vi "compress_discretes_fast_1.vi"(6 "DI state table":T1[](array[typedef]), 8 "discret parameters":bool[](array[boolean]), 9 "DI table":string[](array[string]), 10 "date/time string":string, 11 "table":string) -> (2 "Data to write":bool, 3 "parameters":string)   [LabVIEW 2019, in "PostgreSQL.lvlib"]
uses:
  PostgreSQL.lvlib
  Inputs/Ctl/Parameter State.ctl
  Inputs/Inputs.lvlib
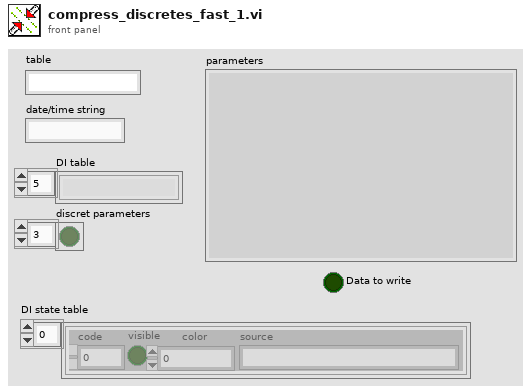
[diagram p1: front panel]
types:
  T1 = typedef "Inputs.lvlib/Parameter State.ctl" = cluster{"code":i32, "visible":bool, "color":u32, "source":string}
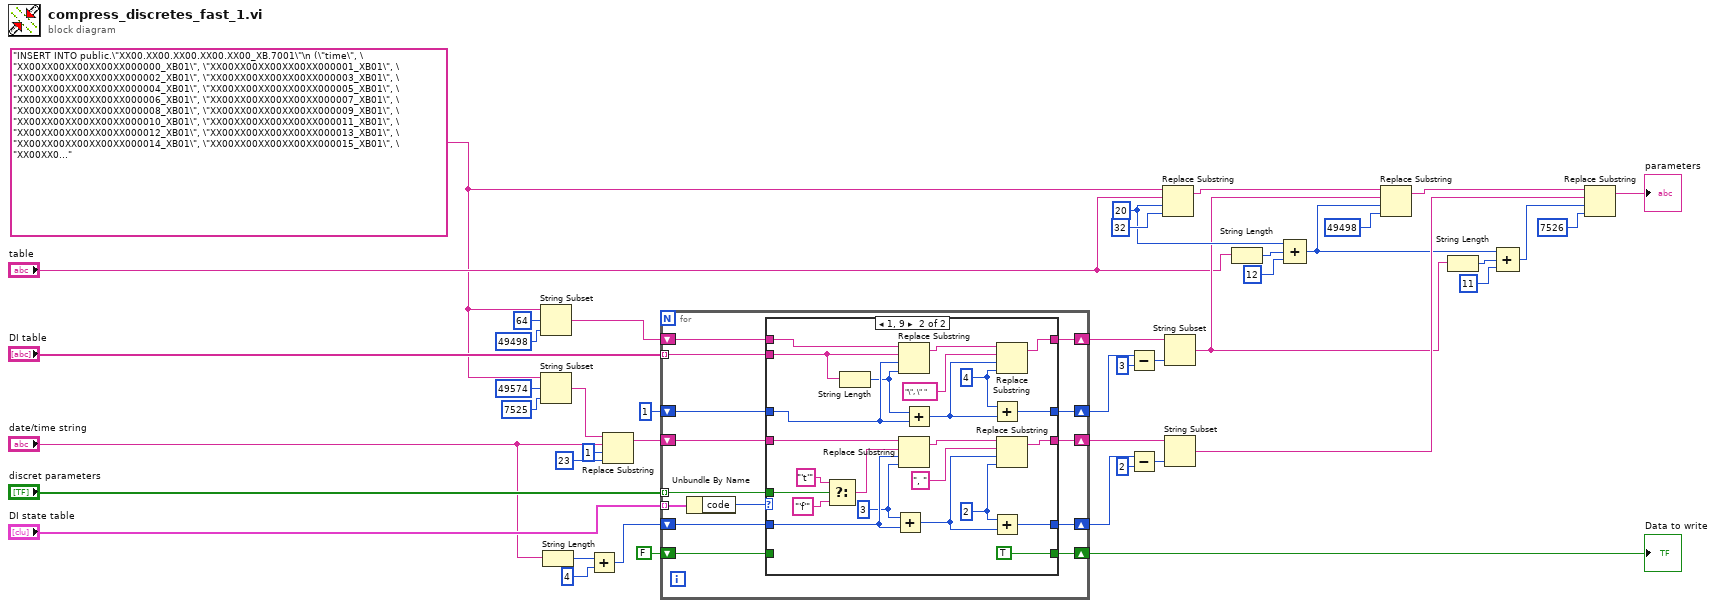
[diagram p0: block diagram]
diagram:
  w32 = 20 ("offset (0)")
  w10 = "INSERT INTO public.\"XX00.XX00.XX00.XX00.XX00_XB.7001\"\n (\"time\", \"XX00XX00XX00XX00XX000000_XB01\", \"XX00XX00XX00XX00XX000001_XB01\", \"XX00XX00XX00XX00XX000002_XB01\", \"XX00XX00XX00XX00XX000003_XB01\", \"XX00XX00XX00XX00XX000004_XB01\", \"XX00XX00XX00XX00XX000005_XB01\", \"XX00XX00XX00XX00XX000006_XB01\", \"XX00XX00XX00XX00XX000007_XB01\", \"XX00XX00XX00XX00XX000008_XB01\", \"XX00XX00XX00XX00XX000009_XB01\", \"XX00XX00XX00XX00XX000010_XB01\", \"XX00XX00XX00XX00XX000011_XB01\", \"XX00XX00XX00XX00XX000012_XB01\", \"XX00XX00XX00XX00XX000013_XB01\", \"XX00XX00XX00XX00XX000014_XB01\", \"XX00XX00XX00XX00XX000015_XB01\", \"XX00XX00XX00XX00XX000016_XB01\", \"XX00XX00XX00XX00XX000017_XB01\", \"XX00XX00XX00XX00XX000018_XB01\", \"XX00XX00XX00XX00XX000019_XB01\", \"XX00XX00XX00XX00XX000020_XB01\", \"XX00XX00XX00XX00XX000021_XB01\", \"XX00XX00XX00XX00XX000022_XB01\", \"XX00XX00XX00XX00XX000023_XB01\", \"XX00XX00XX00XX00XX000024_XB01\", \"XX00XX00XX00XX00XX000025_XB01\", \"XX00XX00XX00XX00XX000026_XB01\", \"XX00XX00XX00XX00XX000027_XB01\", \"XX00XX00XX00XX00XX000028_XB01\", \"XX00XX00XX00XX00XX000029_XB01\", \"XX00XX00XX00XX00XX000030_XB01\", \"XX00XX00XX00XX00XX000031_XB01\", \"XX00XX00XX00XX00XX000032_XB01\", \"XX00XX00XX00XX00XX000033_XB01\", \"XX00XX00XX00XX00XX000034_XB01\", \"XX00XX00XX00XX00XX000035_XB01\", \"XX00XX00XX00XX00XX000036_XB01\", \"XX00XX00XX00XX00XX000037_XB01\", \"XX00XX00XX00XX00XX000038_XB01\", \"XX00XX00XX00XX00XX000039_XB01\", \"XX00XX00XX00XX00XX000040_XB01\", \"XX00XX00XX00XX00XX000041_XB01\", \"XX00XX00XX00XX00XX000042_XB01\", \"XX00XX00XX00XX00XX000043_XB01\", \"XX00XX00XX00XX00XX000044_XB01\", \"XX00XX00XX00XX00XX000045_XB01\", \"XX00XX00XX00XX00XX000046_XB01\", \"XX00XX00XX00XX00XX000047_XB01\", \"XX00XX00XX00XX00XX000048_XB01\", \"XX00XX00XX00XX00XX000049_XB01\", \"XX00XX00XX00XX00XX000050_XB01\", \"XX00XX00XX00XX00XX000051_XB01\", \"XX00XX00XX00XX00XX000052_XB01\", \"XX00XX00XX00XX00XX000053_XB01\", \"XX00XX00XX00XX00XX000054_XB01\", \"XX00XX00XX00XX00XX000055_XB01\", \"XX00XX00XX00XX00XX000056_XB01\", \"XX00XX00XX00XX00XX000057_XB01\", \"XX00XX00XX00XX00XX000058_XB01\", \"XX00XX00XX00XX00XX000059_XB01\", \"XX00XX00XX00XX00XX000060_XB01\", \"XX00XX00XX00XX00XX000061_XB01\", \"XX00XX00XX00XX00XX000062_XB01\", \"XX00XX00XX00XX00XX000063_XB01\", \"XX00XX00XX00XX00XX000064_XB01\", \"XX00XX00XX00XX00XX000065_XB01\", \"XX00XX00XX00XX00XX000066_XB01\", \"XX00XX00XX00XX00XX000067_XB01\", \"XX00XX00XX00XX00XX000068_XB01\", \"XX00XX00XX00XX00XX000069_XB01\", \"XX00XX00XX00XX00XX000070_XB01\", \"XX00XX00XX00XX00XX000071_XB01\", \"XX00XX00XX00XX00XX000072_XB01\", \"XX00XX00XX00XX00XX000073_XB01\", \"XX00XX00XX00XX00XX000074_XB01\", \"XX00XX00XX00XX00XX000075_XB01\", \"XX00XX00XX00XX00XX000076_XB01\", \"XX00XX00XX00XX00XX000077_XB01\", \"XX00XX00XX00XX00XX000078_XB01\", \"XX00XX00XX00XX00XX000079_XB01\", \"XX00XX00XX00XX00XX000080_XB01\", \"XX00XX00XX00XX00XX000081_XB01\", \"XX00XX00XX00XX00XX000082_XB01\", \"XX00XX00XX00XX00XX000083_XB01\", \"XX00XX00XX00XX00XX000084_XB01\", \"XX00XX00XX00XX00XX000085_XB01\", \"XX00XX00XX00XX00XX000086_XB01\", \"XX00XX00XX00XX00XX000087_XB01\", \"XX00XX00XX00XX00XX000088_XB01\", \"XX00XX00XX00XX00XX000089_XB01\", \"XX00XX00XX00XX00XX000090_XB01\", \"XX00XX00XX00XX00XX000091_XB01\", \"XX00XX00XX00XX00XX000092_XB01\", \"XX00XX00XX00XX00XX000093_XB01\", \"XX00XX00XX00XX00XX000094_XB01\", \"XX00XX00XX00XX00XX000095_XB01\", \"XX00XX00XX00XX00XX000096_XB01\", \"XX00XX00XX00XX00XX000097_XB01\", \"XX00XX00XX00XX00XX000098_XB01\", \"XX00XX00XX00XX00XX000099_XB01\", \"XX00XX00XX00XX00XX000100_XB01\", \"XX00XX00XX00XX00XX000101_XB01\", \"XX00XX00XX00XX00XX000102_XB01\", \"XX00XX00XX00XX00XX000103_XB01\", \"XX00XX00XX00XX00XX000104_XB01\", \"XX00XX00XX00XX00XX000105_XB01\", \"XX00XX00XX00XX00XX000106_XB01\", \"XX00XX00XX00XX00XX000107_XB01\", \"XX00XX00XX00XX00XX000108_XB01\", \"XX00XX00XX00XX00XX000109_XB01\", \"XX00XX00XX00XX00XX000110_XB01\", \"XX00XX00XX00XX00XX000111_XB01\", \"XX00XX00XX00XX00XX000112_XB01\", \"XX00XX00XX00XX00XX000113_XB01\", \"XX00XX00XX00XX00XX000114_XB01\", \"XX00XX00XX00XX00XX000115_XB01\", \"XX00XX00XX00XX00XX000116_XB01\", \"XX00XX00XX00XX00XX000117_XB01\", \"XX00XX00XX00XX00XX000118_XB01\", \"XX00XX00XX00XX00XX000119_XB01\", \"XX00XX00XX00XX00XX000120_XB01\", \"XX00XX00XX00XX00XX000121_XB01\", \"XX00XX00XX00XX00XX000122_XB01\", \"XX00XX00XX00XX00XX000123_XB01\", \"XX00XX00XX00XX00XX000124_XB01\", \"XX00XX00XX00XX00XX000125_XB01\", \"XX00XX00XX00XX00XX000126_XB01\", \"XX00XX00XX00XX00XX000127_XB01\", \"XX00XX00XX00XX00XX000128_XB01\", \"XX00XX00XX00XX00XX000129_XB01\", \"XX00XX00XX00XX00XX000130_XB01\", \"XX00XX00XX00XX00XX000131_XB01\", \"XX00XX00XX00XX00XX000132_XB01\", \"XX00XX00XX00XX00XX000133_XB01\", \"XX00XX00XX00XX00XX000134_XB01\", \"XX00XX00XX00XX00XX000135_XB01\", \"XX00XX00XX00XX00XX000136_XB01\", \"XX00XX00XX00XX00XX000137_XB01\", \"XX00XX00XX00XX00XX000138_XB01\", \"XX00XX00XX00XX00XX000139_XB01\", \"XX00XX00XX00XX00XX000140_XB01\", \"XX00XX00XX00XX00XX000141_XB01\", \"XX00XX00XX00XX00XX000142_XB01\", \"XX00XX00XX00XX00XX000143_XB01\", \"XX00XX00XX00XX00XX000144_XB01\", \"XX00XX00XX00XX00XX000145_XB01\", \"XX00XX00XX00XX00XX000146_XB01\", \"XX00XX00XX00XX00XX000147_XB01\", \"XX00XX00XX00XX00XX000148_XB01\", \"XX00XX00XX00XX00XX000149_XB01\", \"XX00XX00XX00XX00XX000150_XB01\", \"XX00XX00XX00XX00XX000151_XB01\", \"XX00XX00XX00XX00XX000152_XB01\", \"XX00XX00XX00XX00XX000153_XB01\", \"XX00XX00XX00XX00XX000154_XB01\", \"XX00XX00XX00XX00XX000155_XB01\", \"XX00XX00XX00XX00XX000156_XB01\", \"XX00XX00XX00XX00XX000157_XB01\", \"XX00XX00XX00XX00XX000158_XB01\", \"XX00XX00XX00XX00XX000159_XB01\", \"XX00XX00XX00XX00XX000160_XB01\", \"XX00XX00XX00XX00XX000161_XB01\", \"XX00XX00XX00XX00XX000162_XB01\", \"XX00XX00XX00XX00XX000163_XB01\", \"XX00XX00XX00XX00XX000164_XB01\", \"XX00XX00XX00XX00XX000165_XB01\", \"XX00XX00XX00XX00XX000166_XB01\", \"XX00XX00XX00XX00XX000167_XB01\", \"XX00XX00XX00XX00XX000168_XB01\", \"XX00XX00XX00XX00XX000169_XB01\", \"XX00XX00XX00XX00XX000170_XB01\", \"XX00XX00XX00XX00XX000171_XB01\", \"XX00XX00XX00XX00XX000172_XB01\", \"XX00XX00XX00XX00XX000173_XB01\", \"XX00XX00XX00XX00XX000174_XB01\", \"XX00XX00XX00XX00XX000175_XB01\", \"XX00XX00XX00XX00XX000176_XB01\", \"XX00XX00XX00XX00XX000177_XB01\", \"XX00XX00XX00XX00XX000178_XB01\", \"XX00XX00XX00XX00XX000179_XB01\", \"XX00XX00XX00XX00XX000180_XB01\", \"XX00XX00XX00XX00XX000181_XB01\", \"XX00XX00XX00XX00XX000182_XB01\", \"XX00XX00XX00XX00XX000183_XB01\", \"XX00XX00XX00XX00XX000184_XB01\", \"XX00XX00XX00XX00XX000185_XB01\", \"XX00XX00XX00XX00XX000186_XB01\", \"XX00XX00XX00XX00XX000187_XB01\", \"XX00XX00XX00XX00XX000188_XB01\", \"XX00XX00XX00XX00XX000189_XB01\", \"XX00XX00XX00XX00XX000190_XB01\", \"XX00XX00XX00XX00XX000191_XB01\", \"XX00XX00XX00XX00XX000192_XB01\", \"XX00XX00XX00XX00XX000193_XB01\", \"XX00XX00XX00XX00XX000194_XB01\", \"XX00XX00XX00XX00XX000195_XB01\", \"XX00XX00XX00XX00XX000196_XB01\", \"XX00XX00XX00XX00XX000197_XB01\", \"XX00XX00XX00XX00XX000198_XB01\", \"XX00XX00XX00XX00XX000199_XB01\", \"XX00XX00XX00XX00XX000200_XB01\", \"XX00XX00XX00XX00XX000201_XB01\", \"XX00XX00XX00XX00XX000202_XB01\", \"XX00XX00XX00XX00XX000203_XB01\", \"XX00XX00XX00XX00XX000204_XB01\", \"XX00XX00XX00XX00XX000205_XB01\", \"XX00XX00XX00XX00XX000206_XB01\", \"XX00XX00XX00XX00XX000207_XB01\", \"XX00XX00XX00XX00XX000208_XB01\", \"XX00XX00XX00XX00XX000209_XB01\", \"XX00XX00XX00XX00XX000210_XB01\", \"XX00XX00XX00XX00XX000211_XB01\", \"XX00XX00XX00XX00XX000212_XB01\", \"XX00XX00XX00XX00XX000213_XB01\", \"XX00XX00XX00XX00XX000214_XB01\", \"XX00XX00XX00XX00XX000215_XB01\", \"XX00XX00XX00XX00XX000216_XB01\", \"XX00XX00XX00XX00XX000217_XB01\", \"XX00XX00XX00XX00XX000218_XB01\", \"XX00XX00XX00XX00XX000219_XB01\", \"XX00XX00XX00XX00XX000220_XB01\", \"XX00XX00XX00XX00XX000221_XB01\", \"XX00XX00XX00XX00XX000222_XB01\", \"XX00XX00XX00XX00XX000223_XB01\", \"XX00XX00XX00XX00XX000224_XB01\", \"XX00XX00XX00XX00XX000225_XB01\", \"XX00XX00XX00XX00XX000226_XB01\", \"XX00XX00XX00XX00XX000227_XB01\", \"XX00XX00XX00XX00XX000228_XB01\", \"XX00XX00XX00XX00XX000229_XB01\", \"XX00XX00XX00XX00XX000230_XB01\", \"XX00XX00XX00XX00XX000231_XB01\", \"XX00XX00XX00XX00XX000232_XB01\", \"XX00XX00XX00XX00XX000233_XB01\", \"XX00XX00XX00XX00XX000234_XB01\", \"XX00XX00XX00XX00XX000235_XB01\", \"XX00XX00XX00XX00XX000236_XB01\", \"XX00XX00XX00XX00XX000237_XB01\", \"XX00XX00XX00XX00XX000238_XB01\", \"XX00XX00XX00XX00XX000239_XB01\", \"XX00XX00XX00XX00XX000240_XB01\", \"XX00XX00XX00XX00XX000241_XB01\", \"XX00XX00XX00XX00XX000242_XB01\", \"XX00XX00XX00XX00XX000243_XB01\", \"XX00XX00XX00XX00XX000244_XB01\", \"XX00XX00XX00XX00XX000245_XB01\", \"XX00XX00XX00XX00XX000246_XB01\", \"XX00XX00XX00XX00XX000247_XB01\", \"XX00XX00XX00XX00XX000248_XB01\", \"XX00XX00XX00XX00XX000249_XB01\", \"XX00XX00XX00XX00XX000250_XB01\", \"XX00XX00XX00XX00XX000251_XB01\", \"XX00XX00XX00XX00XX000252_XB01\", \"XX00XX00XX00XX00XX000253_XB01\", \"XX00XX00XX00XX00XX000254_XB01\", \"XX00XX00XX00XX00XX000255_XB01\", \"XX00XX00XX00XX00XX000256_XB01\", \"XX00XX00XX00XX00XX000257_XB01\", \"XX00XX00XX00XX00XX000258_XB01\", \"XX00XX00XX00XX00XX000259_XB01\", \"XX00XX00XX00XX00XX000260_XB01\", \"XX00XX00XX00XX00XX000261_XB01\", \"XX00XX00XX00XX00XX000262_XB01\", \"XX00XX00XX00XX00XX000263_XB01\", \"XX00XX00XX00XX00XX000264_XB01\", \"XX00XX00XX00XX00XX000265_XB01\", \"XX00XX00XX00XX00XX000266_XB01\", \"XX00XX00XX00XX00XX000267_XB01\", \"XX00XX00XX00XX00XX000268_XB01\", \"XX00XX00XX00XX00XX000269_XB01\", \"XX00XX00XX00XX00XX000270_XB01\", \"XX00XX00XX00XX00XX000271_XB01\", \"XX00XX00XX00XX00XX000272_XB01\", \"XX00XX00XX00XX00XX000273_XB01\", \"XX00XX00XX00XX00XX000274_XB01\", \"XX00XX00XX00XX00XX000275_XB01\", \"XX00XX00XX00XX00XX000276_XB01\", \"XX00XX00XX00XX00XX000277_XB01\", \"XX00XX00XX00XX00XX000278_XB01\", \"XX00XX00XX00XX00XX000279_XB01\", \"XX00XX00XX00XX00XX000280_XB01\", \"XX00XX00XX00XX00XX000281_XB01\", \"XX00XX00XX00XX00XX000282_XB01\", \"XX00XX00XX00XX00XX000283_XB01\", \"XX00XX00XX00XX00XX000284_XB01\", \"XX00XX00XX00XX00XX000285_XB01\", \"XX00XX00XX00XX00XX000286_XB01\", \"XX00XX00XX00XX00XX000287_XB01\", \"XX00XX00XX00XX00XX000288_XB01\", \"XX00XX00XX00XX00XX000289_XB01\", \"XX00XX00XX00XX00XX000290_XB01\", \"XX00XX00XX00XX00XX000291_XB01\", \"XX00XX00XX00XX00XX000292_XB01\", \"XX00XX00XX00XX00XX000293_XB01\", \"XX00XX00XX00XX00XX000294_XB01\", \"XX00XX00XX00XX00XX000295_XB01\", \"XX00XX00XX00XX00XX000296_XB01\", \"XX00XX00XX00XX00XX000297_XB01\", \"XX00XX00XX00XX00XX000298_XB01\", \"XX00XX00XX00XX00XX000299_XB01\", \"XX00XX00XX00XX00XX000300_XB01\", \"XX00XX00XX00XX00XX000301_XB01\", \"XX00XX00XX00XX00XX000302_XB01\", \"XX00XX00XX00XX00XX000303_XB01\", \"XX00XX00XX00XX00XX000304_XB01\", \"XX00XX00XX00XX00XX000305_XB01\", \"XX00XX00XX00XX00XX000306_XB01\", \"XX00XX00XX00XX00XX000307_XB01\", \"XX00XX00XX00XX00XX000308_XB01\", \"XX00XX00XX00XX00XX000309_XB01\", \"XX00XX00XX00XX00XX000310_XB01\", \"XX00XX00XX00XX00XX000311_XB01\", \"XX00XX00XX00XX00XX000312_XB01\", \"XX00XX00XX00XX00XX000313_XB01\", \"XX00XX00XX00XX00XX000314_XB01\", \"XX00XX00XX00XX00XX000315_XB01\", \"XX00XX00XX00XX00XX000316_XB01\", \"XX00XX00XX00XX00XX000317_XB01\", \"XX00XX00XX00XX00XX000318_XB01\", \"XX00XX00XX00XX00XX000319_XB01\", \"XX00XX00XX00XX00XX000320_XB01\", \"XX00XX00XX00XX00XX000321_XB01\", \"XX00XX00XX00XX00XX000322_XB01\", \"XX00XX00XX00XX00XX000323_XB01\", \"XX00XX00XX00XX00XX000324_XB01\", \"XX00XX00XX00XX00XX000325_XB01\", \"XX00XX00XX00XX00XX000326_XB01\", \"XX00XX00XX00XX00XX000327_XB01\", \"XX00XX00XX00XX00XX000328_XB01\", \"XX00XX00XX00XX00XX000329_XB01\", \"XX00XX00XX00XX00XX000330_XB01\", \"XX00XX00XX00XX00XX000331_XB01\", \"XX00XX00XX00XX00XX000332_XB01\", \"XX00XX00XX00XX00XX000333_XB01\", \"XX00XX00XX00XX00XX000334_XB01\", \"XX00XX00XX00XX00XX000335_XB01\", \"XX00XX00XX00XX00XX000336_XB01\", \"XX00XX00XX00XX00XX000337_XB01\", \"XX00XX00XX00XX00XX000338_XB01\", \"XX00XX00XX00XX00XX000339_XB01\", \"XX00XX00XX00XX00XX000340_XB01\", \"XX00XX00XX00XX00XX000341_XB01\", \"XX00XX00XX00XX00XX000342_XB01\", \"XX00XX00XX00XX00XX000343_XB01\", \"XX00XX00XX00XX00XX000344_XB01\", \"XX00XX00XX00XX00XX000345_XB01\", \"XX00XX00XX00XX00XX000346_XB01\", \"XX00XX00XX00XX00XX000347_XB01\", \"XX00XX00XX00XX00XX000348_XB01\", \"XX00XX00XX00XX00XX000349_XB01\", \"XX00XX00XX00XX00XX000350_XB01\", \"XX00XX00XX00XX00XX000351_XB01\", \"XX00XX00XX00XX00XX000352_XB01\", \"XX00XX00XX00XX00XX000353_XB01\", \"XX00XX00XX00XX00XX000354_XB01\", \"XX00XX00XX00XX00XX000355_XB01\", \"XX00XX00XX00XX00XX000356_XB01\", \"XX00XX00XX00XX00XX000357_XB01\", \"XX00XX00XX00XX00XX000358_XB01\", \"XX00XX00XX00XX00XX000359_XB01\", \"XX00XX00XX00XX00XX000360_XB01\", \"XX00XX00XX00XX00XX000361_XB01\", \"XX00XX00XX00XX00XX000362_XB01\", \"XX00XX00XX00XX00XX000363_XB01\", \"XX00XX00XX00XX00XX000364_XB01\", \"XX00XX00XX00XX00XX000365_XB01\", \"XX00XX00XX00XX00XX000366_XB01\", \"XX00XX00XX00XX00XX000367_XB01\", \"XX00XX00XX00XX00XX000368_XB01\", \"XX00XX00XX00XX00XX000369_XB01\", \"XX00XX00XX00XX00XX000370_XB01\", \"XX00XX00XX00XX00XX000371_XB01\", \"XX00XX00XX00XX00XX000372_XB01\", \"XX00XX00XX00XX00XX000373_XB01\", \"XX00XX00XX00XX00XX000374_XB01\", \"XX00XX00XX00XX00XX000375_XB01\", \"XX00XX00XX00XX00XX000376_XB01\", \"XX00XX00XX00XX00XX000377_XB01\", \"XX00XX00XX00XX00XX000378_XB01\", \"XX00XX00XX00XX00XX000379_XB01\", \"XX00XX00XX00XX00XX000380_XB01\", \"XX00XX00XX00XX00XX000381_XB01\", \"XX00XX00XX00XX00XX000382_XB01\", \"XX00XX00XX00XX00XX000383_XB01\", \"XX00XX00XX00XX00XX000384_XB01\", \"XX00XX00XX00XX00XX000385_XB01\", \"XX00XX00XX00XX00XX000386_XB01\", \"XX00XX00XX00XX00XX000387_XB01\", \"XX00XX00XX00XX00XX000388_XB01\", \"XX00XX00XX00XX00XX000389_XB01\", \"XX00XX00XX00XX00XX000390_XB01\", \"XX00XX00XX00XX00XX000391_XB01\", \"XX00XX00XX00XX00XX000392_XB01\", \"XX00XX00XX00XX00XX000393_XB01\", \"XX00XX00XX00XX00XX000394_XB01\", \"XX00XX00XX00XX00XX000395_XB01\", \"XX00XX00XX00XX00XX000396_XB01\", \"XX00XX00XX00XX00XX000397_XB01\", \"XX00XX00XX00XX00XX000398_XB01\", \"XX00XX00XX00XX00XX000399_XB01\", \"XX00XX00XX00XX00XX000400_XB01\", \"XX00XX00XX00XX00XX000401_XB01\", \"XX00XX00XX00XX00XX000402_XB01\", \"XX00XX00XX00XX00XX000403_XB01\", \"XX00XX00XX00XX00XX000404_XB01\", \"XX00XX00XX00XX00XX000405_XB01\", \"XX00XX00XX00XX00XX000406_XB01\", \"XX00XX00XX00XX00XX000407_XB01\", \"XX00XX00XX00XX00XX000408_XB01\", \"XX00XX00XX00XX00XX000409_XB01\", \"XX00XX00XX00XX00XX000410_XB01\", \"XX00XX00XX00XX00XX000411_XB01\", \"XX00XX00XX00XX00XX000412_XB01\", \"XX00XX00XX00XX00XX000413_XB01\", \"XX00XX00XX00XX00XX000414_XB01\", \"XX00XX00XX00XX00XX000415_XB01\", \"XX00XX00XX00XX00XX000416_XB01\", \"XX00XX00XX00XX00XX000417_XB01\", \"XX00XX00XX00XX00XX000418_XB01\", \"XX00XX00XX00XX00XX000419_XB01\", \"XX00XX00XX00XX00XX000420_XB01\", \"XX00XX00XX00XX00XX000421_XB01\", \"XX00XX00XX00XX00XX000422_XB01\", \"XX00XX00XX00XX00XX000423_XB01\", \"XX00XX00XX00XX00XX000424_XB01\", \"XX00XX00XX00XX00XX000425_XB01\", \"XX00XX00XX00XX00XX000426_XB01\", \"XX00XX00XX00XX00XX000427_XB01\", \"XX00XX00XX00XX00XX000428_XB01\", \"XX00XX00XX00XX00XX000429_XB01\", \"XX00XX00XX00XX00XX000430_XB01\", \"XX00XX00XX00XX00XX000431_XB01\", \"XX00XX00XX00XX00XX000432_XB01\", \"XX00XX00XX00XX00XX000433_XB01\", \"XX00XX00XX00XX00XX000434_XB01\", \"XX00XX00XX00XX00XX000435_XB01\", \"XX00XX00XX00XX00XX000436_XB01\", \"XX00XX00XX00XX00XX000437_XB01\", \"XX00XX00XX00XX00XX000438_XB01\", \"XX00XX00XX00XX00XX000439_XB01\", \"XX00XX00XX00XX00XX000440_XB01\", \"XX00XX00XX00XX00XX000441_XB01\", \"XX00XX00XX00XX00XX000442_XB01\", \"XX00XX00XX00XX00XX000443_XB01\", \"XX00XX00XX00XX00XX000444_XB01\", \"XX00XX00XX00XX00XX000445_XB01\", \"XX00XX00XX00XX00XX000446_XB01\", \"XX00XX00XX00XX00XX000447_XB01\", \"XX00XX00XX00XX00XX000448_XB01\", \"XX00XX00XX00XX00XX000449_XB01\", \"XX00XX00XX00XX00XX000450_XB01\", \"XX00XX00XX00XX00XX000451_XB01\", \"XX00XX00XX00XX00XX000452_XB01\", \"XX00XX00XX00XX00XX000453_XB01\", \"XX00XX00XX00XX00XX000454_XB01\", \"XX00XX00XX00XX00XX000455_XB01\", \"XX00XX00XX00XX00XX000456_XB01\", \"XX00XX00XX00XX00XX000457_XB01\", \"XX00XX00XX00XX00XX000458_XB01\", \"XX00XX00XX00XX00XX000459_XB01\", \"XX00XX00XX00XX00XX000460_XB01\", \"XX00XX00XX00XX00XX000461_XB01\", \"XX00XX00XX00XX00XX000462_XB01\", \"XX00XX00XX00XX00XX000463_XB01\", \"XX00XX00XX00XX00XX000464_XB01\", \"XX00XX00XX00XX00XX000465_XB01\", \"XX00XX00XX00XX00XX000466_XB01\", \"XX00XX00XX00XX00XX000467_XB01\", \"XX00XX00XX00XX00XX000468_XB01\", \"XX00XX00XX00XX00XX000469_XB01\", \"XX00XX00XX00XX00XX000470_XB01\", \"XX00XX00XX00XX00XX000471_XB01\", \"XX00XX00XX00XX00XX000472_XB01\", \"XX00XX00XX00XX00XX000473_XB01\", \"XX00XX00XX00XX00XX000474_XB01\", \"XX00XX00XX00XX00XX000475_XB01\", \"XX00XX00XX00XX00XX000476_XB01\", \"XX00XX00XX00XX00XX000477_XB01\", \"XX00XX00XX00XX00XX000478_XB01\", \"XX00XX00XX00XX00XX000479_XB01\", \"XX00XX00XX00XX00XX000480_XB01\", \"XX00XX00XX00XX00XX000481_XB01\", \"XX00XX00XX00XX00XX000482_XB01\", \"XX00XX00XX00XX00XX000483_XB01\", \"XX00XX00XX00XX00XX000484_XB01\", \"XX00XX00XX00XX00XX000485_XB01\", \"XX00XX00XX00XX00XX000486_XB01\", \"XX00XX00XX00XX00XX000487_XB01\", \"XX00XX00XX00XX00XX000488_XB01\", \"XX00XX00XX00XX00XX000489_XB01\", \"XX00XX00XX00XX00XX000490_XB01\", \"XX00XX00XX00XX00XX000491_XB01\", \"XX00XX00XX00XX00XX000492_XB01\", \"XX00XX00XX00XX00XX000493_XB01\", \"XX00XX00XX00XX00XX000494_XB01\", \"XX00XX00XX00XX00XX000495_XB01\", \"XX00XX00XX00XX00XX000496_XB01\", \"XX00XX00XX00XX00XX000497_XB01\", \"XX00XX00XX00XX00XX000498_XB01\", \"XX00XX00XX00XX00XX000499_XB01\", \"XX00XX00XX00XX00XX000500_XB01\", \"XX00XX00XX00XX00XX000501_XB01\", \"XX00XX00XX00XX00XX000502_XB01\", \"XX00XX00XX00XX00XX000503_XB01\", \"XX00XX00XX00XX00XX000504_XB01\", \"XX00XX00XX00XX00XX000505_XB01\", \"XX00XX00XX00XX00XX000506_XB01\", \"XX00XX00XX00XX00XX000507_XB01\", \"XX00XX00XX00XX00XX000508_XB01\", \"XX00XX00XX00XX00XX000509_XB01\", \"XX00XX00XX00XX00XX000510_XB01\", \"XX00XX00XX00XX00XX000511_XB01\", \"XX00XX00XX00XX00XX000512_XB01\", \"XX00XX00XX00XX00XX000513_XB01\", \"XX00XX00XX00XX00XX000514_XB01\", \"XX00XX00XX00XX00XX000515_XB01\", \"XX00XX00XX00XX00XX000516_XB01\", \"XX00XX00XX00XX00XX000517_XB01\", \"XX00XX00XX00XX00XX000518_XB01\", \"XX00XX00XX00XX00XX000519_XB01\", \"XX00XX00XX00XX00XX000520_XB01\", \"XX00XX00XX00XX00XX000521_XB01\", \"XX00XX00XX00XX00XX000522_XB01\", \"XX00XX00XX00XX00XX000523_XB01\", \"XX00XX00XX00XX00XX000524_XB01\", \"XX00XX00XX00XX00XX000525_XB01\", \"XX00XX00XX00XX00XX000526_XB01\", \"XX00XX00XX00XX00XX000527_XB01\", \"XX00XX00XX00XX00XX000528_XB01\", \"XX00XX00XX00XX00XX000529_XB01\", \"XX00XX00XX00XX00XX000530_XB01\", \"XX00XX00XX00XX00XX000531_XB01\", \"XX00XX00XX00XX00XX000532_XB01\", \"XX00XX00XX00XX00XX000533_XB01\", \"XX00XX00XX00XX00XX000534_XB01\", \"XX00XX00XX00XX00XX000535_XB01\", \"XX00XX00XX00XX00XX000536_XB01\", \"XX00XX00XX00XX00XX000537_XB01\", \"XX00XX00XX00XX00XX000538_XB01\", \"XX00XX00XX00XX00XX000539_XB01\", \"XX00XX00XX00XX00XX000540_XB01\", \"XX00XX00XX00XX00XX000541_XB01\", \"XX00XX00XX00XX00XX000542_XB01\", \"XX00XX00XX00XX00XX000543_XB01\", \"XX00XX00XX00XX00XX000544_XB01\", \"XX00XX00XX00XX00XX000545_XB01\", \"XX00XX00XX00XX00XX000546_XB01\", \"XX00XX00XX00XX00XX000547_XB01\", \"XX00XX00XX00XX00XX000548_XB01\", \"XX00XX00XX00XX00XX000549_XB01\", \"XX00XX00XX00XX00XX000550_XB01\", \"XX00XX00XX00XX00XX000551_XB01\", \"XX00XX00XX00XX00XX000552_XB01\", \"XX00XX00XX00XX00XX000553_XB01\", \"XX00XX00XX00XX00XX000554_XB01\", \"XX00XX00XX00XX00XX000555_XB01\", \"XX00XX00XX00XX00XX000556_XB01\", \"XX00XX00XX00XX00XX000557_XB01\", \"XX00XX00XX00XX00XX000558_XB01\", \"XX00XX00XX00XX00XX000559_XB01\", \"XX00XX00XX00XX00XX000560_XB01\", \"XX00XX00XX00XX00XX000561_XB01\", \"XX00XX00XX00XX00XX000562_XB01\", \"XX00XX00XX00XX00XX000563_XB01\", \"XX00XX00XX00XX00XX000564_XB01\", \"XX00XX00XX00XX00XX000565_XB01\", \"XX00XX00XX00XX00XX000566_XB01\", \"XX00XX00XX00XX00XX000567_XB01\", \"XX00XX00XX00XX00XX000568_XB01\", \"XX00XX00XX00XX00XX000569_XB01\", \"XX00XX00XX00XX00XX000570_XB01\", \"XX00XX00XX00XX00XX000571_XB01\", \"XX00XX00XX00XX00XX000572_XB01\", \"XX00XX00XX00XX00XX000573_XB01\", \"XX00XX00XX00XX00XX000574_XB01\", \"XX00XX00XX00XX00XX000575_XB01\", \"XX00XX00XX00XX00XX000576_XB01\", \"XX00XX00XX00XX00XX000577_XB01\", \"XX00XX00XX00XX00XX000578_XB01\", \"XX00XX00XX00XX00XX000579_XB01\", \"XX00XX00XX00XX00XX000580_XB01\", \"XX00XX00XX00XX00XX000581_XB01\", \"XX00XX00XX00XX00XX000582_XB01\", \"XX00XX00XX00XX00XX000583_XB01\", \"XX00XX00XX00XX00XX000584_XB01\", \"XX00XX00XX00XX00XX000585_XB01\", \"XX00XX00XX00XX00XX000586_XB01\", \"XX00XX00XX00XX00XX000587_XB01\", \"XX00XX00XX00XX00XX000588_XB01\", \"XX00XX00XX00XX00XX000589_XB01\", \"XX00XX00XX00XX00XX000590_XB01\", \"XX00XX00XX00XX00XX000591_XB01\", \"XX00XX00XX00XX00XX000592_XB01\", \"XX00XX00XX00XX00XX000593_XB01\", \"XX00XX00XX00XX00XX000594_XB01\", \"XX00XX00XX00XX00XX000595_XB01\", \"XX00XX00XX00XX00XX000596_XB01\", \"XX00XX00XX00XX00XX000597_XB01\", \"XX00XX00XX00XX00XX000598_XB01\", \"XX00XX00XX00XX00XX000599_XB01\", \"XX00XX00XX00XX00XX000600_XB01\", \"XX00XX00XX00XX00XX000601_XB01\", \"XX00XX00XX00XX00XX000602_XB01\", \"XX00XX00XX00XX00XX000603_XB01\", \"XX00XX00XX00XX00XX000604_XB01\", \"XX00XX00XX00XX00XX000605_XB01\", \"XX00XX00XX00XX00XX000606_XB01\", \"XX00XX00XX00XX00XX000607_XB01\", \"XX00XX00XX00XX00XX000608_XB01\", \"XX00XX00XX00XX00XX000609_XB01\", \"XX00XX00XX00XX00XX000610_XB01\", \"XX00XX00XX00XX00XX000611_XB01\", \"XX00XX00XX00XX00XX000612_XB01\", \"XX00XX00XX00XX00XX000613_XB01\", \"XX00XX00XX00XX00XX000614_XB01\", \"XX00XX00XX00XX00XX000615_XB01\", \"XX00XX00XX00XX00XX000616_XB01\", \"XX00XX00XX00XX00XX000617_XB01\", \"XX00XX00XX00XX00XX000618_XB01\", \"XX00XX00XX00XX00XX000619_XB01\", \"XX00XX00XX00XX00XX000620_XB01\", \"XX00XX00XX00XX00XX000621_XB01\", \"XX00XX00XX00XX00XX000622_XB01\", \"XX00XX00XX00XX00XX000623_XB01\", \"XX00XX00XX00XX00XX000624_XB01\", \"XX00XX00XX00XX00XX000625_XB01\", \"XX00XX00XX00XX00XX000626_XB01\", \"XX00XX00XX00XX00XX000627_XB01\", \"XX00XX00XX00XX00XX000628_XB01\", \"XX00XX00XX00XX00XX000629_XB01\", \"XX00XX00XX00XX00XX000630_XB01\", \"XX00XX00XX00XX00XX000631_XB01\", \"XX00XX00XX00XX00XX000632_XB01\", \"XX00XX00XX00XX00XX000633_XB01\", \"XX00XX00XX00XX00XX000634_XB01\", \"XX00XX00XX00XX00XX000635_XB01\", \"XX00XX00XX00XX00XX000636_XB01\", \"XX00XX00XX00XX00XX000637_XB01\", \"XX00XX00XX00XX00XX000638_XB01\", \"XX00XX00XX00XX00XX000639_XB01\", \"XX00XX00XX00XX00XX000640_XB01\", \"XX00XX00XX00XX00XX000641_XB01\", \"XX00XX00XX00XX00XX000642_XB01\", \"XX00XX00XX00XX00XX000643_XB01\", \"XX00XX00XX00XX00XX000644_XB01\", \"XX00XX00XX00XX00XX000645_XB01\", \"XX00XX00XX00XX00XX000646_XB01\", \"XX00XX00XX00XX00XX000647_XB01\", \"XX00XX00XX00XX00XX000648_XB01\", \"XX00XX00XX00XX00XX000649_XB01\", \"XX00XX00XX00XX00XX000650_XB01\", \"XX00XX00XX00XX00XX000651_XB01\", \"XX00XX00XX00XX00XX000652_XB01\", \"XX00XX00XX00XX00XX000653_XB01\", \"XX00XX00XX00XX00XX000654_XB01\", \"XX00XX00XX00XX00XX000655_XB01\", \"XX00XX00XX00XX00XX000656_XB01\", \"XX00XX00XX00XX00XX000657_XB01\", \"XX00XX00XX00XX00XX000658_XB01\", \"XX00XX00XX00XX00XX000659_XB01\", \"XX00XX00XX00XX00XX000660_XB01\", \"XX00XX00XX00XX00XX000661_XB01\", \"XX00XX00XX00XX00XX000662_XB01\", \"XX00XX00XX00XX00XX000663_XB01\", \"XX00XX00XX00XX00XX000664_XB01\", \"XX00XX00XX00XX00XX000665_XB01\", \"XX00XX00XX00XX00XX000666_XB01\", \"XX00XX00XX00XX00XX000667_XB01\", \"XX00XX00XX00XX00XX000668_XB01\", \"XX00XX00XX00XX00XX000669_XB01\", \"XX00XX00XX00XX00XX000670_XB01\", \"XX00XX00XX00XX00XX000671_XB01\", \"XX00XX00XX00XX00XX000672_XB01\", \"XX00XX00XX00XX00XX000673_XB01\", \"XX00XX00XX00XX00XX000674_XB01\", \"XX00XX00XX00XX00XX000675_XB01\", \"XX00XX00XX00XX00XX000676_XB01\", \"XX00XX00XX00XX00XX000677_XB01\", \"XX00XX00XX00XX00XX000678_XB01\", \"XX00XX00XX00XX00XX000679_XB01\", \"XX00XX00XX00XX00XX000680_XB01\", \"XX00XX00XX00XX00XX000681_XB01\", \"XX00XX00XX00XX00XX000682_XB01\", \"XX00XX00XX00XX00XX000683_XB01\", \"XX00XX00XX00XX00XX000684_XB01\", \"XX00XX00XX00XX00XX000685_XB01\", \"XX00XX00XX00XX00XX000686_XB01\", \"XX00XX00XX00XX00XX000687_XB01\", \"XX00XX00XX00XX00XX000688_XB01\", \"XX00XX00XX00XX00XX000689_XB01\", \"XX00XX00XX00XX00XX000690_XB01\", \"XX00XX00XX00XX00XX000691_XB01\", \"XX00XX00XX00XX00XX000692_XB01\", \"XX00XX00XX00XX00XX000693_XB01\", \"XX00XX00XX00XX00XX000694_XB01\", \"XX00XX00XX00XX00XX000695_XB01\", \"XX00XX00XX00XX00XX000696_XB01\", \"XX00XX00XX00XX00XX000697_XB01\", \"XX00XX00XX00XX00XX000698_XB01\", \"XX00XX00XX00XX00XX000699_XB01\", \"XX00XX00XX00XX00XX000700_XB01\", \"XX00XX00XX00XX00XX000701_XB01\", \"XX00XX00XX00XX00XX000702_XB01\", \"XX00XX00XX00XX00XX000703_XB01\", \"XX00XX00XX00XX00XX000704_XB01\", \"XX00XX00XX00XX00XX000705_XB01\", \"XX00XX00XX00XX00XX000706_XB01\", \"XX00XX00XX00XX00XX000707_XB01\", \"XX00XX00XX00XX00XX000708_XB01\", \"XX00XX00XX00XX00XX000709_XB01\", \"XX00XX00XX00XX00XX000710_XB01\", \"XX00XX00XX00XX00XX000711_XB01\", \"XX00XX00XX00XX00XX000712_XB01\", \"XX00XX00XX00XX00XX000713_XB01\", \"XX00XX00XX00XX00XX000714_XB01\", \"XX00XX00XX00XX00XX000715_XB01\", \"XX00XX00XX00XX00XX000716_XB01\", \"XX00XX00XX00XX00XX000717_XB01\", \"XX00XX00XX00XX00XX000718_XB01\", \"XX00XX00XX00XX00XX000719_XB01\", \"XX00XX00XX00XX00XX000720_XB01\", \"XX00XX00XX00XX00XX000721_XB01\", \"XX00XX00XX00XX00XX000722_XB01\", \"XX00XX00XX00XX00XX000723_XB01\", \"XX00XX00XX00XX00XX000724_XB01\", \"XX00XX00XX00XX00XX000725_XB01\", \"XX00XX00XX00XX00XX000726_XB01\", \"XX00XX00XX00XX00XX000727_XB01\", \"XX00XX00XX00XX00XX000728_XB01\", \"XX00XX00XX00XX00XX000729_XB01\", \"XX00XX00XX00XX00XX000730_XB01\", \"XX00XX00XX00XX00XX000731_XB01\", \"XX00XX00XX00XX00XX000732_XB01\", \"XX00XX00XX00XX00XX000733_XB01\", \"XX00XX00XX00XX00XX000734_XB01\", \"XX00XX00XX00XX00XX000735_XB01\", \"XX00XX00XX00XX00XX000736_XB01\", \"XX00XX00XX00XX00XX000737_XB01\", \"XX00XX00XX00XX00XX000738_XB01\", \"XX00XX00XX00XX00XX000739_XB01\", \"XX00XX00XX00XX00XX000740_XB01\", \"XX00XX00XX00XX00XX000741_XB01\", \"XX00XX00XX00XX00XX000742_XB01\", \"XX00XX00XX00XX00XX000743_XB01\", \"XX00XX00XX00XX00XX000744_XB01\", \"XX00XX00XX00XX00XX000745_XB01\", \"XX00XX00XX00XX00XX000746_XB01\", \"XX00XX00XX00XX00XX000747_XB01\", \"XX00XX00XX00XX00XX000748_XB01\", \"XX00XX00XX00XX00XX000749_XB01\", \"XX00XX00XX00XX00XX000750_XB01\", \"XX00XX00XX00XX00XX000751_XB01\", \"XX00XX00XX00XX00XX000752_XB01\", \"XX00XX00XX00XX00XX000753_XB01\", \"XX00XX00XX00XX00XX000754_XB01\", \"XX00XX00XX00XX00XX000755_XB01\", \"XX00XX00XX00XX00XX000756_XB01\", \"XX00XX00XX00XX00XX000757_XB01\", \"XX00XX00XX00XX00XX000758_XB01\", \"XX00XX00XX00XX00XX000759_XB01\", \"XX00XX00XX00XX00XX000760_XB01\", \"XX00XX00XX00XX00XX000761_XB01\", \"XX00XX00XX00XX00XX000762_XB01\", \"XX00XX00XX00XX00XX000763_XB01\", \"XX00XX00XX00XX00XX000764_XB01\", \"XX00XX00XX00XX00XX000765_XB01\", \"XX00XX00XX00XX00XX000766_XB01\", \"XX00XX00XX00XX00XX000767_XB01\", \"XX00XX00XX00XX00XX000768_XB01\", \"XX00XX00XX00XX00XX000769_XB01\", \"XX00XX00XX00XX00XX000770_XB01\", \"XX00XX00XX00XX00XX000771_XB01\", \"XX00XX00XX00XX00XX000772_XB01\", \"XX00XX00XX00XX00XX000773_XB01\", \"XX00XX00XX00XX00XX000774_XB01\", \"XX00XX00XX00XX00XX000775_XB01\", \"XX00XX00XX00XX00XX000776_XB01\", \"XX00XX00XX00XX00XX000777_XB01\", \"XX00XX00XX00XX00XX000778_XB01\", \"XX00XX00XX00XX00XX000779_XB01\", \"XX00XX00XX00XX00XX000780_XB01\", \"XX00XX00XX00XX00XX000781_XB01\", \"XX00XX00XX00XX00XX000782_XB01\", \"XX00XX00XX00XX00XX000783_XB01\", \"XX00XX00XX00XX00XX000784_XB01\", \"XX00XX00XX00XX00XX000785_XB01\", \"XX00XX00XX00XX00XX000786_XB01\", \"XX00XX00XX00XX00XX000787_XB01\", \"XX00XX00XX00XX00XX000788_XB01\", \"XX00XX00XX00XX00XX000789_XB01\", \"XX00XX00XX00XX00XX000790_XB01\", \"XX00XX00XX00XX00XX000791_XB01\", \"XX00XX00XX00XX00XX000792_XB01\", \"XX00XX00XX00XX00XX000793_XB01\", \"XX00XX00XX00XX00XX000794_XB01\", \"XX00XX00XX00XX00XX000795_XB01\", \"XX00XX00XX00XX00XX000796_XB01\", \"XX00XX00XX00XX00XX000797_XB01\", \"XX00XX00XX00XX00XX000798_XB01\", \"XX00XX00XX00XX00XX000799_XB01\", \"XX00XX00XX00XX00XX000800_XB01\", \"XX00XX00XX00XX00XX000801_XB01\", \"XX00XX00XX00XX00XX000802_XB01\", \"XX00XX00XX00XX00XX000803_XB01\", \"XX00XX00XX00XX00XX000804_XB01\", \"XX00XX00XX00XX00XX000805_XB01\", \"XX00XX00XX00XX00XX000806_XB01\", \"XX00XX00XX00XX00XX000807_XB01\", \"XX00XX00XX00XX00XX000808_XB01\", \"XX00XX00XX00XX00XX000809_XB01\", \"XX00XX00XX00XX00XX000810_XB01\", \"XX00XX00XX00XX00XX000811_XB01\", \"XX00XX00XX00XX00XX000812_XB01\", \"XX00XX00XX00XX00XX000813_XB01\", \"XX00XX00XX00XX00XX000814_XB01\", \"XX00XX00XX00XX00XX000815_XB01\", \"XX00XX00XX00XX00XX000816_XB01\", \"XX00XX00XX00XX00XX000817_XB01\", \"XX00XX00XX00XX00XX000818_XB01\", \"XX00XX00XX00XX00XX000819_XB01\", \"XX00XX00XX00XX00XX000820_XB01\", \"XX00XX00XX00XX00XX000821_XB01\", \"XX00XX00XX00XX00XX000822_XB01\", \"XX00XX00XX00XX00XX000823_XB01\", \"XX00XX00XX00XX00XX000824_XB01\", \"XX00XX00XX00XX00XX000825_XB01\", \"XX00XX00XX00XX00XX000826_XB01\", \"XX00XX00XX00XX00XX000827_XB01\", \"XX00XX00XX00XX00XX000828_XB01\", \"XX00XX00XX00XX00XX000829_XB01\", \"XX00XX00XX00XX00XX000830_XB01\", \"XX00XX00XX00XX00XX000831_XB01\", \"XX00XX00XX00XX00XX000832_XB01\", \"XX00XX00XX00XX00XX000833_XB01\", \"XX00XX00XX00XX00XX000834_XB01\", \"XX00XX00XX00XX00XX000835_XB01\", \"XX00XX00XX00XX00XX000836_XB01\", \"XX00XX00XX00XX00XX000837_XB01\", \"XX00XX00XX00XX00XX000838_XB01\", \"XX00XX00XX00XX00XX000839_XB01\", \"XX00XX00XX00XX00XX000840_XB01\", \"XX00XX00XX00XX00XX000841_XB01\", \"XX00XX00XX00XX00XX000842_XB01\", \"XX00XX00XX00XX00XX000843_XB01\", \"XX00XX00XX00XX00XX000844_XB01\", \"XX00XX00XX00XX00XX000845_XB01\", \"XX00XX00XX00XX00XX000846_XB01\", \"XX00XX00XX00XX00XX000847_XB01\", \"XX00XX00XX00XX00XX000848_XB01\", \"XX00XX00XX00XX00XX000849_XB01\", \"XX00XX00XX00XX00XX000850_XB01\", \"XX00XX00XX00XX00XX000851_XB01\", \"XX00XX00XX00XX00XX000852_XB01\", \"XX00XX00XX00XX00XX000853_XB01\", \"XX00XX00XX00XX00XX000854_XB01\", \"XX00XX00XX00XX00XX000855_XB01\", \"XX00XX00XX00XX00XX000856_XB01\", \"XX00XX00XX00XX00XX000857_XB01\", \"XX00XX00XX00XX00XX000858_XB01\", \"XX00XX00XX00XX00XX000859_XB01\", \"XX00XX00XX00XX00XX000860_XB01\", \"XX00XX00XX00XX00XX000861_XB01\", \"XX00XX00XX00XX00XX000862_XB01\", \"XX00XX00XX00XX00XX000863_XB01\", \"XX00XX00XX00XX00XX000864_XB01\", \"XX00XX00XX00XX00XX000865_XB01\", \"XX00XX00XX00XX00XX000866_XB01\", \"XX00XX00XX00XX00XX000867_XB01\", \"XX00XX00XX00XX00XX000868_XB01\", \"XX00XX00XX00XX00XX000869_XB01\", \"XX00XX00XX00XX00XX000870_XB01\", \"XX00XX00XX00XX00XX000871_XB01\", \"XX00XX00XX00XX00XX000872_XB01\", \"XX00XX00XX00XX00XX000873_XB01\", \"XX00XX00XX00XX00XX000874_XB01\", \"XX00XX00XX00XX00XX000875_XB01\", \"XX00XX00XX00XX00XX000876_XB01\", \"XX00XX00XX00XX00XX000877_XB01\", \"XX00XX00XX00XX00XX000878_XB01\", \"XX00XX00XX00XX00XX000879_XB01\", \"XX00XX00XX00XX00XX000880_XB01\", \"XX00XX00XX00XX00XX000881_XB01\", \"XX00XX00XX00XX00XX000882_XB01\", \"XX00XX00XX00XX00XX000883_XB01\", \"XX00XX00XX00XX00XX000884_XB01\", \"XX00XX00XX00XX00XX000885_XB01\", \"XX00XX00XX00XX00XX000886_XB01\", \"XX00XX00XX00XX00XX000887_XB01\", \"XX00XX00XX00XX00XX000888_XB01\", \"XX00XX00XX00XX00XX000889_XB01\", \"XX00XX00XX00XX00XX000890_XB01\", \"XX00XX00XX00XX00XX000891_XB01\", \"XX00XX00XX00XX00XX000892_XB01\", \"XX00XX00XX00XX00XX000893_XB01\", \"XX00XX00XX00XX00XX000894_XB01\", \"XX00XX00XX00XX00XX000895_XB01\", \"XX00XX00XX00XX00XX000896_XB01\", \"XX00XX00XX00XX00XX000897_XB01\", \"XX00XX00XX00XX00XX000898_XB01\", \"XX00XX00XX00XX00XX000899_XB01\", \"XX00XX00XX00XX00XX000900_XB01\", \"XX00XX00XX00XX00XX000901_XB01\", \"XX00XX00XX00XX00XX000902_XB01\", \"XX00XX00XX00XX00XX000903_XB01\", \"XX00XX00XX00XX00XX000904_XB01\", \"XX00XX00XX00XX00XX000905_XB01\", \"XX00XX00XX00XX00XX000906_XB01\", \"XX00XX00XX00XX00XX000907_XB01\", \"XX00XX00XX00XX00XX000908_XB01\", \"XX00XX00XX00XX00XX000909_XB01\", \"XX00XX00XX00XX00XX000910_XB01\", \"XX00XX00XX00XX00XX000911_XB01\", \"XX00XX00XX00XX00XX000912_XB01\", \"XX00XX00XX00XX00XX000913_XB01\", \"XX00XX00XX00XX00XX000914_XB01\", \"XX00XX00XX00XX00XX000915_XB01\", \"XX00XX00XX00XX00XX000916_XB01\", \"XX00XX00XX00XX00XX000917_XB01\", \"XX00XX00XX00XX00XX000918_XB01\", \"XX00XX00XX00XX00XX000919_XB01\", \"XX00XX00XX00XX00XX000920_XB01\", \"XX00XX00XX00XX00XX000921_XB01\", \"XX00XX00XX00XX00XX000922_XB01\", \"XX00XX00XX00XX00XX000923_XB01\", \"XX00XX00XX00XX00XX000924_XB01\", \"XX00XX00XX00XX00XX000925_XB01\", \"XX00XX00XX00XX00XX000926_XB01\", \"XX00XX00XX00XX00XX000927_XB01\", \"XX00XX00XX00XX00XX000928_XB01\", \"XX00XX00XX00XX00XX000929_XB01\", \"XX00XX00XX00XX00XX000930_XB01\", \"XX00XX00XX00XX00XX000931_XB01\", \"XX00XX00XX00XX00XX000932_XB01\", \"XX00XX00XX00XX00XX000933_XB01\", \"XX00XX00XX00XX00XX000934_XB01\", \"XX00XX00XX00XX00XX000935_XB01\", \"XX00XX00XX00XX00XX000936_XB01\", \"XX00XX00XX00XX00XX000937_XB01\", \"XX00XX00XX00XX00XX000938_XB01\", \"XX00XX00XX00XX00XX000939_XB01\", \"XX00XX00XX00XX00XX000940_XB01\", \"XX00XX00XX00XX00XX000941_XB01\", \"XX00XX00XX00XX00XX000942_XB01\", \"XX00XX00XX00XX00XX000943_XB01\", \"XX00XX00XX00XX00XX000944_XB01\", \"XX00XX00XX00XX00XX000945_XB01\", \"XX00XX00XX00XX00XX000946_XB01\", \"XX00XX00XX00XX00XX000947_XB01\", \"XX00XX00XX00XX00XX000948_XB01\", \"XX00XX00XX00XX00XX000949_XB01\", \"XX00XX00XX00XX00XX000950_XB01\", \"XX00XX00XX00XX00XX000951_XB01\", \"XX00XX00XX00XX00XX000952_XB01\", \"XX00XX00XX00XX00XX000953_XB01\", \"XX00XX00XX00XX00XX000954_XB01\", \"XX00XX00XX00XX00XX000955_XB01\", \"XX00XX00XX00XX00XX000956_XB01\", \"XX00XX00XX00XX00XX000957_XB01\", \"XX00XX00XX00XX00XX000958_XB01\", \"XX00XX00XX00XX00XX000959_XB01\", \"XX00XX00XX00XX00XX000960_XB01\", \"XX00XX00XX00XX00XX000961_XB01\", \"XX00XX00XX00XX00XX000962_XB01\", \"XX00XX00XX00XX00XX000963_XB01\", \"XX00XX00XX00XX00XX000964_XB01\", \"XX00XX00XX00XX00XX000965_XB01\", \"XX00XX00XX00XX00XX000966_XB01\", \"XX00XX00XX00XX00XX000967_XB01\", \"XX00XX00XX00XX00XX000968_XB01\", \"XX00XX00XX00XX00XX000969_XB01\", \"XX00XX00XX00XX00XX000970_XB01\", \"XX00XX00XX00XX00XX000971_XB01\", \"XX00XX00XX00XX00XX000972_XB01\", \"XX00XX00XX00XX00XX000973_XB01\", \"XX00XX00XX00XX00XX000974_XB01\", \"XX00XX00XX00XX00XX000975_XB01\", \"XX00XX00XX00XX00XX000976_XB01\", \"XX00XX00XX00XX00XX000977_XB01\", \"XX00XX00XX00XX00XX000978_XB01\", \"XX00XX00XX00XX00XX000979_XB01\", \"XX00XX00XX00XX00XX000980_XB01\", \"XX00XX00XX00XX00XX000981_XB01\", \"XX00XX00XX00XX00XX000982_XB01\", \"XX00XX00XX00XX00XX000983_XB01\", \"XX00XX00XX00XX00XX000984_XB01\", \"XX00XX00XX00XX00XX000985_XB01\", \"XX00XX00XX00XX00XX000986_XB01\", \"XX00XX00XX00XX00XX000987_XB01\", \"XX00XX00XX00XX00XX000988_XB01\", \"XX00XX00XX00XX00XX000989_XB01\", \"XX00XX00XX00XX00XX000990_XB01\", \"XX00XX00XX00XX00XX000991_XB01\", \"XX00XX00XX00XX00XX000992_XB01\", \"XX00XX00XX00XX00XX000993_XB01\", \"XX00XX00XX00XX00XX000994_XB01\", \"XX00XX00XX00XX00XX000995_XB01\", \"XX00XX00XX00XX00XX000996_XB01\", \"XX00XX00XX00XX00XX000997_XB01\", \"XX00XX00XX00XX00XX000998_XB01\", \"XX00XX00XX00XX00XX000999_XB01\", \"XX00XX00XX00XX00XX001000_XB01\", \"XX00XX00XX00XX00XX001001_XB01\", \"XX00XX00XX00XX00XX001002_XB01\", \"XX00XX00XX00XX00XX001003_XB01\", \"XX00XX00XX00XX00XX001004_XB01\", \"XX00XX00XX00XX00XX001005_XB01\", \"XX00XX00XX00XX00XX001006_XB01\", \"XX00XX00XX00XX00XX001007_XB01\", \"XX00XX00XX00XX00XX001008_XB01\", \"XX00XX00XX00XX00XX001009_XB01\", \"XX00XX00XX00XX00XX001010_XB01\", \"XX00XX00XX00XX00XX001011_XB01\", \"XX00XX00XX00XX00XX001012_XB01\", \"XX00XX00XX00XX00XX001013_XB01\", \"XX00XX00XX00XX00XX001014_XB01\", \"XX00XX00XX00XX00XX001015_XB01\", \"XX00XX00XX00XX00XX001016_XB01\", \"XX00XX00XX00XX00XX001017_XB01\", \"XX00XX00XX00XX00XX001018_XB01\", \"XX00XX00XX00XX00XX001019_XB01\", \"XX00XX00XX00XX00XX001020_XB01\", \"XX00XX00XX00XX00XX001021_XB01\", \"XX00XX00XX00XX00XX001022_XB01\", \"XX00XX00XX00XX00XX001023_XB01\", \"XX00XX00XX00XX00XX001024_XB01\", \"XX00XX00XX00XX00XX001025_XB01\", \"XX00XX00XX00XX00XX001026_XB01\", \"XX00XX00XX00XX00XX001027_XB01\", \"XX00XX00XX00XX00XX001028_XB01\", \"XX00XX00XX00XX00XX001029_XB01\", \"XX00XX00XX00XX00XX001030_XB01\", \"XX00XX00XX00XX00XX001031_XB01\", \"XX00XX00XX00XX00XX001032_XB01\", \"XX00XX00XX00XX00XX001033_XB01\", \"XX00XX00XX00XX00XX001034_XB01\", \"XX00XX00XX00XX00XX001035_XB01\", \"XX00XX00XX00XX00XX001036_XB01\", \"XX00XX00XX00XX00XX001037_XB01\", \"XX00XX00XX00XX00XX001038_XB01\", \"XX00XX00XX00XX00XX001039_XB01\", \"XX00XX00XX00XX00XX001040_XB01\", \"XX00XX00XX00XX00XX001041_XB01\", \"XX00XX00XX00XX00XX001042_XB01\", \"XX00XX00XX00XX00XX001043_XB01\", \"XX00XX00XX00XX00XX001044_XB01\", \"XX00XX00XX00XX00XX001045_XB01\", \"XX00XX00XX00XX00XX001046_XB01\", \"XX00XX00XX00XX00XX001047_XB01\", \"XX00XX00XX00XX00XX001048_XB01\", \"XX00XX00XX00XX00XX001049_XB01\", \"XX00XX00XX00XX00XX001050_XB01\", \"XX00XX00XX00XX00XX001051_XB01\", \"XX00XX00XX00XX00XX001052_XB01\", \"XX00XX00XX00XX00XX001053_XB01\", \"XX00XX00XX00XX00XX001054_XB01\", \"XX00XX00XX00XX00XX001055_XB01\", \"XX00XX00XX00XX00XX001056_XB01\", \"XX00XX00XX00XX00XX001057_XB01\", \"XX00XX00XX00XX00XX001058_XB01\", \"XX00XX00XX00XX00XX001059_XB01\", \"XX00XX00XX00XX00XX001060_XB01\", \"XX00XX00XX00XX00XX001061_XB01\", \"XX00XX00XX00XX00XX001062_XB01\", \"XX00XX00XX00XX00XX001063_XB01\", \"XX00XX00XX00XX00XX001064_XB01\", \"XX00XX00XX00XX00XX001065_XB01\", \"XX00XX00XX00XX00XX001066_XB01\", \"XX00XX00XX00XX00XX001067_XB01\", \"XX00XX00XX00XX00XX001068_XB01\", \"XX00XX00XX00XX00XX001069_XB01\", \"XX00XX00XX00XX00XX001070_XB01\", \"XX00XX00XX00XX00XX001071_XB01\", \"XX00XX00XX00XX00XX001072_XB01\", \"XX00XX00XX00XX00XX001073_XB01\", \"XX00XX00XX00XX00XX001074_XB01\", \"XX00XX00XX00XX00XX001075_XB01\", \"XX00XX00XX00XX00XX001076_XB01\", \"XX00XX00XX00XX00XX001077_XB01\", \"XX00XX00XX00XX00XX001078_XB01\", \"XX00XX00XX00XX00XX001079_XB01\", \"XX00XX00XX00XX00XX001080_XB01\", \"XX00XX00XX00XX00XX001081_XB01\", \"XX00XX00XX00XX00XX001082_XB01\", \"XX00XX00XX00XX00XX001083_XB01\", \"XX00XX00XX00XX00XX001084_XB01\", \"XX00XX00XX00XX00XX001085_XB01\", \"XX00XX00XX00XX00XX001086_XB01\", \"XX00XX00XX00XX00XX001087_XB01\", \"XX00XX00XX00XX00XX001088_XB01\", \"XX00XX00XX00XX00XX001089_XB01\", \"XX00XX00XX00XX00XX001090_XB01\", \"XX00XX00XX00XX00XX001091_XB01\", \"XX00XX00XX00XX00XX001092_XB01\", \"XX00XX00XX00XX00XX001093_XB01\", \"XX00XX00XX00XX00XX001094_XB01\", \"XX00XX00XX00XX00XX001095_XB01\", \"XX00XX00XX00XX00XX001096_XB01\", \"XX00XX00XX00XX00XX001097_XB01\", \"XX00XX00XX00XX00XX001098_XB01\", \"XX00XX00XX00XX00XX001099_XB01\", \"XX00XX00XX00XX00XX001100_XB01\", \"XX00XX00XX00XX00XX001101_XB01\", \"XX00XX00XX00XX00XX001102_XB01\", \"XX00XX00XX00XX00XX001103_XB01\", \"XX00XX00XX00XX00XX001104_XB01\", \"XX00XX00XX00XX00XX001105_XB01\", \"XX00XX00XX00XX00XX001106_XB01\", \"XX00XX00XX00XX00XX001107_XB01\", \"XX00XX00XX00XX00XX001108_XB01\", \"XX00XX00XX00XX00XX001109_XB01\", \"XX00XX00XX00XX00XX001110_XB01\", \"XX00XX00XX00XX00XX001111_XB01\", \"XX00XX00XX00XX00XX001112_XB01\", \"XX00XX00XX00XX00XX001113_XB01\", \"XX00XX00XX00XX00XX001114_XB01\", \"XX00XX00XX00XX00XX001115_XB01\", \"XX00XX00XX00XX00XX001116_XB01\", \"XX00XX00XX00XX00XX001117_XB01\", \"XX00XX00XX00XX00XX001118_XB01\", \"XX00XX00XX00XX00XX001119_XB01\", \"XX00XX00XX00XX00XX001120_XB01\", \"XX00XX00XX00XX00XX001121_XB01\", \"XX00XX00XX00XX00XX001122_XB01\", \"XX00XX00XX00XX00XX001123_XB01\", \"XX00XX00XX00XX00XX001124_XB01\", \"XX00XX00XX00XX00XX001125_XB01\", \"XX00XX00XX00XX00XX001126_XB01\", \"XX00XX00XX00XX00XX001127_XB01\", \"XX00XX00XX00XX00XX001128_XB01\", \"XX00XX00XX00XX00XX001129_XB01\", \"XX00XX00XX00XX00XX001130_XB01\", \"XX00XX00XX00XX00XX001131_XB01\", \"XX00XX00XX00XX00XX001132_XB01\", \"XX00XX00XX00XX00XX001133_XB01\", \"XX00XX00XX00XX00XX001134_XB01\", \"XX00XX00XX00XX00XX001135_XB01\", \"XX00XX00XX00XX00XX001136_XB01\", \"XX00XX00XX00XX00XX001137_XB01\", \"XX00XX00XX00XX00XX001138_XB01\", \"XX00XX00XX00XX00XX001139_XB01\", \"XX00XX00XX00XX00XX001140_XB01\", \"XX00XX00XX00XX00XX001141_XB01\", \"XX00XX00XX00XX00XX001142_XB01\", \"XX00XX00XX00XX00XX001143_XB01\", \"XX00XX00XX00XX00XX001144_XB01\", \"XX00XX00XX00XX00XX001145_XB01\", \"XX00XX00XX00XX00XX001146_XB01\", \"XX00XX00XX00XX00XX001147_XB01\", \"XX00XX00XX00XX00XX001148_XB01\", \"XX00XX00XX00XX00XX001149_XB01\", \"XX00XX00XX00XX00XX001150_XB01\", \"XX00XX00XX00XX00XX001151_XB01\", \"XX00XX00XX00XX00XX001152_XB01\", \"XX00XX00XX00XX00XX001153_XB01\", \"XX00XX00XX00XX00XX001154_XB01\", \"XX00XX00XX00XX00XX001155_XB01\", \"XX00XX00XX00XX00XX001156_XB01\", \"XX00XX00XX00XX00XX001157_XB01\", \"XX00XX00XX00XX00XX001158_XB01\", \"XX00XX00XX00XX00XX001159_XB01\", \"XX00XX00XX00XX00XX001160_XB01\", \"XX00XX00XX00XX00XX001161_XB01\", \"XX00XX00XX00XX00XX001162_XB01\", \"XX00XX00XX00XX00XX001163_XB01\", \"XX00XX00XX00XX00XX001164_XB01\", \"XX00XX00XX00XX00XX001165_XB01\", \"XX00XX00XX00XX00XX001166_XB01\", \"XX00XX00XX00XX00XX001167_XB01\", \"XX00XX00XX00XX00XX001168_XB01\", \"XX00XX00XX00XX00XX001169_XB01\", \"XX00XX00XX00XX00XX001170_XB01\", \"XX00XX00XX00XX00XX001171_XB01\", \"XX00XX00XX00XX00XX001172_XB01\", \"XX00XX00XX00XX00XX001173_XB01\", \"XX00XX00XX00XX00XX001174_XB01\", \"XX00XX00XX00XX00XX001175_XB01\", \"XX00XX00XX00XX00XX001176_XB01\", \"XX00XX00XX00XX00XX001177_XB01\", \"XX00XX00XX00XX00XX001178_XB01\", \"XX00XX00XX00XX00XX001179_XB01\", \"XX00XX00XX00XX00XX001180_XB01\", \"XX00XX00XX00XX00XX001181_XB01\", \"XX00XX00XX00XX00XX001182_XB01\", \"XX00XX00XX00XX00XX001183_XB01\", \"XX00XX00XX00XX00XX001184_XB01\", \"XX00XX00XX00XX00XX001185_XB01\", \"XX00XX00XX00XX00XX001186_XB01\", \"XX00XX00XX00XX00XX001187_XB01\", \"XX00XX00XX00XX00XX001188_XB01\", \"XX00XX00XX00XX00XX001189_XB01\", \"XX00XX00XX00XX00XX001190_XB01\", \"XX00XX00XX00XX00XX001191_XB01\", \"XX00XX00XX00XX00XX001192_XB01\", \"XX00XX00XX00XX00XX001193_XB01\", \"XX00XX00XX00XX00XX001194_XB01\", \"XX00XX00XX00XX00XX001195_XB01\", \"XX00XX00XX00XX00XX001196_XB01\", \"XX00XX00XX00XX00XX001197_XB01\", \"XX00XX00XX00XX00XX001198_XB01\", \"XX00XX00XX00XX00XX001199_XB01\", \"XX00XX00XX00XX00XX001200_XB01\", \"XX00XX00XX00XX00XX001201_XB01\", \"XX00XX00XX00XX00XX001202_XB01\", \"XX00XX00XX00XX00XX001203_XB01\", \"XX00XX00XX00XX00XX001204_XB01\", \"XX00XX00XX00XX00XX001205_XB01\", \"XX00XX00XX00XX00XX001206_XB01\", \"XX00XX00XX00XX00XX001207_XB01\", \"XX00XX00XX00XX00XX001208_XB01\", \"XX00XX00XX00XX00XX001209_XB01\", \"XX00XX00XX00XX00XX001210_XB01\", \"XX00XX00XX00XX00XX001211_XB01\", \"XX00XX00XX00XX00XX001212_XB01\", \"XX00XX00XX00XX00XX001213_XB01\", \"XX00XX00XX00XX00XX001214_XB01\", \"XX00XX00XX00XX00XX001215_XB01\", \"XX00XX00XX00XX00XX001216_XB01\", \"XX00XX00XX00XX00XX001217_XB01\", \"XX00XX00XX00XX00XX001218_XB01\", \"XX00XX00XX00XX00XX001219_XB01\", \"XX00XX00XX00XX00XX001220_XB01\", \"XX00XX00XX00XX00XX001221_XB01\", \"XX00XX00XX00XX00XX001222_XB01\", \"XX00XX00XX00XX00XX001223_XB01\", \"XX00XX00XX00XX00XX001224_XB01\", \"XX00XX00XX00XX00XX001225_XB01\", \"XX00XX00XX00XX00XX001226_XB01\", \"XX00XX00XX00XX00XX001227_XB01\", \"XX00XX00XX00XX00XX001228_XB01\", \"XX00XX00XX00XX00XX001229_XB01\", \"XX00XX00XX00XX00XX001230_XB01\", \"XX00XX00XX00XX00XX001231_XB01\", \"XX00XX00XX00XX00XX001232_XB01\", \"XX00XX00XX00XX00XX001233_XB01\", \"XX00XX00XX00XX00XX001234_XB01\", \"XX00XX00XX00XX00XX001235_XB01\", \"XX00XX00XX00XX00XX001236_XB01\", \"XX00XX00XX00XX00XX001237_XB01\", \"XX00XX00XX00XX00XX001238_XB01\", \"XX00XX00XX00XX00XX001239_XB01\", \"XX00XX00XX00XX00XX001240_XB01\", \"XX00XX00XX00XX00XX001241_XB01\", \"XX00XX00XX00XX00XX001242_XB01\", \"XX00XX00XX00XX00XX001243_XB01\", \"XX00XX00XX00XX00XX001244_XB01\", \"XX00XX00XX00XX00XX001245_XB01\", \"XX00XX00XX00XX00XX001246_XB01\", \"XX00XX00XX00XX00XX001247_XB01\", \"XX00XX00XX00XX00XX001248_XB01\", \"XX00XX00XX00XX00XX001249_XB01\", \"XX00XX00XX00XX00XX001250_XB01\", \"XX00XX00XX00XX00XX001251_XB01\", \"XX00XX00XX00XX00XX001252_XB01\", \"XX00XX00XX00XX00XX001253_XB01\", \"XX00XX00XX00XX00XX001254_XB01\", \"XX00XX00XX00XX00XX001255_XB01\", \"XX00XX00XX00XX00XX001256_XB01\", \"XX00XX00XX00XX00XX001257_XB01\", \"XX00XX00XX00XX00XX001258_XB01\", \"XX00XX00XX00XX00XX001259_XB01\", \"XX00XX00XX00XX00XX001260_XB01\", \"XX00XX00XX00XX00XX001261_XB01\", \"XX00XX00XX00XX00XX001262_XB01\", \"XX00XX00XX00XX00XX001263_XB01\", \"XX00XX00XX00XX00XX001264_XB01\", \"XX00XX00XX00XX00XX001265_XB01\", \"XX00XX00XX00XX00XX001266_XB01\", \"XX00XX00XX00XX00XX001267_XB01\", \"XX00XX00XX00XX00XX001268_XB01\", \"XX00XX00XX00XX00XX001269_XB01\", \"XX00XX00XX00XX00XX001270_XB01\", \"XX00XX00XX00XX00XX001271_XB01\", \"XX00XX00XX00XX00XX001272_XB01\", \"XX00XX00XX00XX00XX001273_XB01\", \"XX00XX00XX00XX00XX001274_XB01\", \"XX00XX00XX00XX00XX001275_XB01\", \"XX00XX00XX00XX00XX001276_XB01\", \"XX00XX00XX00XX00XX001277_XB01\", \"XX00XX00XX00XX00XX001278_XB01\", \"XX00XX00XX00XX00XX001279_XB01\", \"XX00XX00XX00XX00XX001280_XB01\", \"XX00XX00XX00XX00XX001281_XB01\", \"XX00XX00XX00XX00XX001282_XB01\", \"XX00XX00XX00XX00XX001283_XB01\", \"XX00XX00XX00XX00XX001284_XB01\", \"XX00XX00XX00XX00XX001285_XB01\", \"XX00XX00XX00XX00XX001286_XB01\", \"XX00XX00XX00XX00XX001287_XB01\", \"XX00XX00XX00XX00XX001288_XB01\", \"XX00XX00XX00XX00XX001289_XB01\", \"XX00XX00XX00XX00XX001290_XB01\", \"XX00XX00XX00XX00XX001291_XB01\", \"XX00XX00XX00XX00XX001292_XB01\", \"XX00XX00XX00XX00XX001293_XB01\", \"XX00XX00XX00XX00XX001294_XB01\", \"XX00XX00XX00XX00XX001295_XB01\", \"XX00XX00XX00XX00XX001296_XB01\", \"XX00XX00XX00XX00XX001297_XB01\", \"XX00XX00XX00XX00XX001298_XB01\", \"XX00XX00XX00XX00XX001299_XB01\", \"XX00XX00XX00XX00XX001300_XB01\", \"XX00XX00XX00XX00XX001301_XB01\", \"XX00XX00XX00XX00XX001302_XB01\", \"XX00XX00XX00XX00XX001303_XB01\", \"XX00XX00XX00XX00XX001304_XB01\", \"XX00XX00XX00XX00XX001305_XB01\", \"XX00XX00XX00XX00XX001306_XB01\", \"XX00XX00XX00XX00XX001307_XB01\", \"XX00XX00XX00XX00XX001308_XB01\", \"XX00XX00XX00XX00XX001309_XB01\", \"XX00XX00XX00XX00XX001310_XB01\", \"XX00XX00XX00XX00XX001311_XB01\", \"XX00XX00XX00XX00XX001312_XB01\", \"XX00XX00XX00XX00XX001313_XB01\", \"XX00XX00XX00XX00XX001314_XB01\", \"XX00XX00XX00XX00XX001315_XB01\", \"XX00XX00XX00XX00XX001316_XB01\", \"XX00XX00XX00XX00XX001317_XB01\", \"XX00XX00XX00XX00XX001318_XB01\", \"XX00XX00XX00XX00XX001319_XB01\", \"XX00XX00XX00XX00XX001320_XB01\", \"XX00XX00XX00XX00XX001321_XB01\", \"XX00XX00XX00XX00XX001322_XB01\", \"XX00XX00XX00XX00XX001323_XB01\", \"XX00XX00XX00XX00XX001324_XB01\", \"XX00XX00XX00XX00XX001325_XB01\", \"XX00XX00XX00XX00XX001326_XB01\", \"XX00XX00XX00XX00XX001327_XB01\", \"XX00XX00XX00XX00XX001328_XB01\", \"XX00XX00XX00XX00XX001329_XB01\", \"XX00XX00XX00XX00XX001330_XB01\", \"XX00XX00XX00XX00XX001331_XB01\", \"XX00XX00XX00XX00XX001332_XB01\", \"XX00XX00XX00XX00XX001333_XB01\", \"XX00XX00XX00XX00XX001334_XB01\", \"XX00XX00XX00XX00XX001335_XB01\", \"XX00XX00XX00XX00XX001336_XB01\", \"XX00XX00XX00XX00XX001337_XB01\", \"XX00XX00XX00XX00XX001338_XB01\", \"XX00XX00XX00XX00XX001339_XB01\", \"XX00XX00XX00XX00XX001340_XB01\", \"XX00XX00XX00XX00XX001341_XB01\", \"XX00XX00XX00XX00XX001342_XB01\", \"XX00XX00XX00XX00XX001343_XB01\", \"XX00XX00XX00XX00XX001344_XB01\", \"XX00XX00XX00XX00XX001345_XB01\", \"XX00XX00XX00XX00XX001346_XB01\", \"XX00XX00XX00XX00XX001347_XB01\", \"XX00XX00XX00XX00XX001348_XB01\", \"XX00XX00XX00XX00XX001349_XB01\", \"XX00XX00XX00XX00XX001350_XB01\", \"XX00XX00XX00XX00XX001351_XB01\", \"XX00XX00XX00XX00XX001352_XB01\", \"XX00XX00XX00XX00XX001353_XB01\", \"XX00XX00XX00XX00XX001354_XB01\", \"XX00XX00XX00XX00XX001355_XB01\", \"XX00XX00XX00XX00XX001356_XB01\", \"XX00XX00XX00XX00XX001357_XB01\", \"XX00XX00XX00XX00XX001358_XB01\", \"XX00XX00XX00XX00XX001359_XB01\", \"XX00XX00XX00XX00XX001360_XB01\", \"XX00XX00XX00XX00XX001361_XB01\", \"XX00XX00XX00XX00XX001362_XB01\", \"XX00XX00XX00XX00XX001363_XB01\", \"XX00XX00XX00XX00XX001364_XB01\", \"XX00XX00XX00XX00XX001365_XB01\", \"XX00XX00XX00XX00XX001366_XB01\", \"XX00XX00XX00XX00XX001367_XB01\", \"XX00XX00XX00XX00XX001368_XB01\", \"XX00XX00XX00XX00XX001369_XB01\", \"XX00XX00XX00XX00XX001370_XB01\", \"XX00XX00XX00XX00XX001371_XB01\", \"XX00XX00XX00XX00XX001372_XB01\", \"XX00XX00XX00XX00XX001373_XB01\", \"XX00XX00XX00XX00XX001374_XB01\", \"XX00XX00XX00XX00XX001375_XB01\", \"XX00XX00XX00XX00XX001376_XB01\", \"XX00XX00XX00XX00XX001377_XB01\", \"XX00XX00XX00XX00XX001378_XB01\", \"XX00XX00XX00XX00XX001379_XB01\", \"XX00XX00XX00XX00XX001380_XB01\", \"XX00XX00XX00XX00XX001381_XB01\", \"XX00XX00XX00XX00XX001382_XB01\", \"XX00XX00XX00XX00XX001383_XB01\", \"XX00XX00XX00XX00XX001384_XB01\", \"XX00XX00XX00XX00XX001385_XB01\", \"XX00XX00XX00XX00XX001386_XB01\", \"XX00XX00XX00XX00XX001387_XB01\", \"XX00XX00XX00XX00XX001388_XB01\", \"XX00XX00XX00XX00XX001389_XB01\", \"XX00XX00XX00XX00XX001390_XB01\", \"XX00XX00XX00XX00XX001391_XB01\", \"XX00XX00XX00XX00XX001392_XB01\", \"XX00XX00XX00XX00XX001393_XB01\", \"XX00XX00XX00XX00XX001394_XB01\", \"XX00XX00XX00XX00XX001395_XB01\", \"XX00XX00XX00XX00XX001396_XB01\", \"XX00XX00XX00XX00XX001397_XB01\", \"XX00XX00XX00XX00XX001398_XB01\", \"XX00XX00XX00XX00XX001399_XB01\", \"XX00XX00XX00XX00XX001400_XB01\", \"XX00XX00XX00XX00XX001401_XB01\", \"XX00XX00XX00XX00XX001402_XB01\", \"XX00XX00XX00XX00XX001403_XB01\", \"XX00XX00XX00XX00XX001404_XB01\", \"XX00XX00XX00XX00XX001405_XB01\", \"XX00XX00XX00XX00XX001406_XB01\", \"XX00XX00XX00XX00XX001407_XB01\", \"XX00XX00XX00XX00XX001408_XB01\", \"XX00XX00XX00XX00XX001409_XB01\", \"XX00XX00XX00XX00XX001410_XB01\", \"XX00XX00XX00XX00XX001411_XB01\", \"XX00XX00XX00XX00XX001412_XB01\", \"XX00XX00XX00XX00XX001413_XB01\", \"XX00XX00XX00XX00XX001414_XB01\", \"XX00XX00XX00XX00XX001415_XB01\", \"XX00XX00XX00XX00XX001416_XB01\", \"XX00XX00XX00XX00XX001417_XB01\", \"XX00XX00XX00XX00XX001418_XB01\", \"XX00XX00XX00XX00XX001419_XB01\", \"XX00XX00XX00XX00XX001420_XB01\", \"XX00XX00XX00XX00XX001421_XB01\", \"XX00XX00XX00XX00XX001422_XB01\", \"XX00XX00XX00XX00XX001423_XB01\", \"XX00XX00XX00XX00XX001424_XB01\", \"XX00XX00XX00XX00XX001425_XB01\", \"XX00XX00XX00XX00XX001426_XB01\", \"XX00XX00XX00XX00XX001427_XB01\", \"XX00XX00XX00XX00XX001428_XB01\", \"XX00XX00XX00XX00XX001429_XB01\", \"XX00XX00XX00XX00XX001430_XB01\", \"XX00XX00XX00XX00XX001431_XB01\", \"XX00XX00XX00XX00XX001432_XB01\", \"XX00XX00XX00XX00XX001433_XB01\", \"XX00XX00XX00XX00XX001434_XB01\", \"XX00XX00XX00XX00XX001435_XB01\", \"XX00XX00XX00XX00XX001436_XB01\", \"XX00XX00XX00XX00XX001437_XB01\", \"XX00XX00XX00XX00XX001438_XB01\", \"XX00XX00XX00XX00XX001439_XB01\", \"XX00XX00XX00XX00XX001440_XB01\", \"XX00XX00XX00XX00XX001441_XB01\", \"XX00XX00XX00XX00XX001442_XB01\", \"XX00XX00XX00XX00XX001443_XB01\", \"XX00XX00XX00XX00XX001444_XB01\", \"XX00XX00XX00XX00XX001445_XB01\", \"XX00XX00XX00XX00XX001446_XB01\", \"XX00XX00XX00XX00XX001447_XB01\", \"XX00XX00XX00XX00XX001448_XB01\", \"XX00XX00XX00XX00XX001449_XB01\", \"XX00XX00XX00XX00XX001450_XB01\", \"XX00XX00XX00XX00XX001451_XB01\", \"XX00XX00XX00XX00XX001452_XB01\", \"XX00XX00XX00XX00XX001453_XB01\", \"XX00XX00XX00XX00XX001454_XB01\", \"XX00XX00XX00XX00XX001455_XB01\", \"XX00XX00XX00XX00XX001456_XB01\", \"XX00XX00XX00XX00XX001457_XB01\", \"XX00XX00XX00XX00XX001458_XB01\", \"XX00XX00XX00XX00XX001459_XB01\", \"XX00XX00XX00XX00XX001460_XB01\", \"XX00XX00XX00XX00XX001461_XB01\", \"XX00XX00XX00XX00XX001462_XB01\", \"XX00XX00XX00XX00XX001463_XB01\", \"XX00XX00XX00XX00XX001464_XB01\", \"XX00XX00XX00XX00XX001465_XB01\", \"XX00XX00XX00XX00XX001466_XB01\", \"XX00XX00XX00XX00XX001467_XB01\", \"XX00XX00XX00XX00XX001468_XB01\", \"XX00XX00XX00XX00XX001469_XB01\", \"XX00XX00XX00XX00XX001470_XB01\", \"XX00XX00XX00XX00XX001471_XB01\", \"XX00XX00XX00XX00XX001472_XB01\", \"XX00XX00XX00XX00XX001473_XB01\", \"XX00XX00XX00XX00XX001474_XB01\", \"XX00XX00XX00XX00XX001475_XB01\", \"XX00XX00XX00XX00XX001476_XB01\", \"XX00XX00XX00XX00XX001477_XB01\", \"XX00XX00XX00XX00XX001478_XB01\", \"XX00XX00XX00XX00XX001479_XB01\", \"XX00XX00XX00XX00XX001480_XB01\", \"XX00XX00XX00XX00XX001481_XB01\", \"XX00XX00XX00XX00XX001482_XB01\", \"XX00XX00XX00XX00XX001483_XB01\", \"XX00XX00XX00XX00XX001484_XB01\", \"XX00XX00XX00XX00XX001485_XB01\", \"XX00XX00XX00XX00XX001486_XB01\", \"XX00XX00XX00XX00XX001487_XB01\", \"XX00XX00XX00XX00XX001488_XB01\", \"XX00XX00XX00XX00XX001489_XB01\", \"XX00XX00XX00XX00XX001490_XB01\", \"XX00XX00XX00XX00XX001491_XB01\", \"XX00XX00XX00XX00XX001492_XB01\", \"XX00XX00XX00XX00XX001493_XB01\", \"XX00XX00XX00XX00XX001494_XB01\", \"XX00XX00XX00XX00XX001495_XB01\", \"XX00XX00XX00XX00XX001496_XB01\", \"XX00XX00XX00XX00XX001497_XB01\", \"XX00XX00XX00XX00XX001498_XB01\", \"XX00XX00XX00XX00XX001499_XB01\") \nVALUES ( '2017-11-07 12:04:06.000', 'f', 'f', 'f', 'f', 'f', 'f', 'f', 'f', 'f', 'f', 'f', 'f', 'f', 'f', 'f', 'f', 'f', 'f', 'f', 'f', 'f', 'f', 'f', 'f', 'f', 'f', 'f', 'f', 'f', 'f', 'f', 'f', 'f', 'f', 'f', 'f', 'f', 'f', 'f', 'f', 'f', 'f', 'f', 'f', 'f', 'f', 'f', 'f', 'f', 'f', 'f', 'f', 'f', 'f', 'f', 'f', 'f', 'f', 'f', 'f', 'f', 'f', 'f', 'f', 'f', 'f', 'f', 'f', 'f', 'f', 'f', 'f', 'f', 'f', 'f', 'f', 'f', 'f', 'f', 'f', 'f', 'f', 'f', 'f', 'f', 'f', 'f', 'f', 'f', 'f', 'f', 'f', 'f', 'f', 'f', 'f', 'f', 'f', 'f', 'f', 'f', 'f', 'f', 'f', 'f', 'f', 'f', 'f', 'f', 'f', 'f', 'f', 'f', 'f', 'f', 'f', 'f', 'f', 'f', 'f', 'f', 'f', 'f', 'f', 'f', 'f', 'f', 'f', 'f', 'f', 'f', 'f', 'f', 'f', 'f', 'f', 'f', 'f', 'f', 'f', 'f', 'f', 'f', 'f', 'f', 'f', 'f', 'f', 'f', 'f', 'f', 'f', 'f', 'f', 'f', 'f', 'f', 'f', 'f', 'f', 'f', 'f', 'f', 'f', 'f', 'f', 'f', 'f', 'f', 'f', 'f', 'f', 'f', 'f', 'f', 'f', 'f', 'f', 'f', 'f', 'f', 'f', 'f', 'f', 'f', 'f', 'f', 'f', 'f', 'f', 'f', 'f', 'f', 'f', 'f', 'f', 'f', 'f', 'f', 'f', 'f', 'f', 'f', 'f', 'f', 'f', 'f', 'f', 'f', 'f', 'f', 'f', 'f', 'f', 'f', 'f', 'f', 'f', 'f', 'f', 'f', 'f', 'f', 'f', 'f', 'f', 'f', 'f', 'f', 'f', 'f', 'f', 'f', 'f', 'f', 'f', 'f', 'f', 'f', 'f', 'f', 'f', 'f', 'f', 'f', 'f', 'f', 'f', 'f', 'f', 'f', 'f', 'f', 'f', 'f', 'f', 'f', 'f', 'f', 'f', 'f', 'f', 'f', 'f', 'f', 'f', 'f', 'f', 'f', 'f', 'f', 'f', 'f', 'f', 'f', 'f', 'f', 'f', 'f', 'f', 'f', 'f', 'f', 'f', 'f', 'f', 'f', 'f', 'f', 'f', 'f', 'f', 'f', 'f', 'f', 'f', 'f', 'f', 'f', 'f', 'f', 'f', 'f', 'f', 'f', 'f', 'f', 'f', 'f', 'f', 'f', 'f', 'f', 'f', 'f', 'f', 'f', 'f', 'f', 'f', 'f', 'f', 'f', 'f', 'f', 'f', 'f', 'f', 'f', 'f', 'f', 'f', 'f', 'f', 'f', 'f', 'f', 'f', 'f', 'f', 'f', 'f', 'f', 'f', 'f', 'f', 'f', 'f', 'f', 'f', 'f', 'f', 'f', 'f', 'f', 'f', 'f', 'f', 'f', 'f', 'f', 'f', 'f', 'f', 'f', 'f', 'f', 'f', 'f', 'f', 'f', 'f', 'f', 'f', 'f', 'f', 'f', 'f', 'f', 'f', 'f', 'f', 'f', 'f', 'f', 'f', 'f', 'f', 'f', 'f', 'f', 'f', 'f', 'f', 'f', 'f', 'f', 'f', 'f', 'f', 'f', 'f', 'f', 'f', 'f', 'f', 'f', 'f', 'f', 'f', 'f', 'f', 'f', 'f', 'f', 'f', 'f', 'f', 'f', 'f', 'f', 'f', 'f', 'f', 'f', 'f', 'f', 'f', 'f', 'f', 'f', 'f', 'f', 'f', 'f', 'f', 'f', 'f', 'f', 'f', 'f', 'f', 'f', 'f', 'f', 'f', 'f', 'f', 'f', 'f', 'f', 'f', 'f', 'f', 'f', 'f', 'f', 'f', 'f', 'f', 'f', 'f', 'f', 'f', 'f', 'f', 'f', 'f', 'f', 'f', 'f', 'f', 'f', 'f', 'f', 'f', 'f', 'f', 'f', 'f', 'f', 'f', 'f', 'f', 'f', 'f', 'f', 'f', 'f', 'f', 'f', 'f', 'f', 'f', 'f', 'f', 'f', 'f', 'f', 'f', 'f', 'f', 'f', 'f', 'f', 'f', 'f', 'f', 'f', 'f', 'f', 'f', 'f', 'f', 'f', 'f', 'f', 'f', 'f', 'f', 'f', 'f', 'f', 'f', 'f', 'f', 'f', 'f', 'f', 'f', 'f', 'f', 'f', 'f', 'f', 'f', 'f', 'f', 'f', 'f', 'f', 'f', 'f', 'f', 'f', 'f', 'f', 'f', 'f', 'f', 'f', 'f', 'f', 'f', 'f', 'f', 'f', 'f', 'f', 'f', 'f', 'f', 'f', 'f', 'f', 'f', 'f', 'f', 'f', 'f', 'f', 'f', 'f', 'f', 'f', 'f', 'f', 'f', 'f', 'f', 'f', 'f', 'f', 'f', 'f', 'f', 'f', 'f', 'f', 'f', 'f', 'f', 'f', 'f', 'f', 'f', 'f', 'f', 'f', 'f', 'f', 'f', 'f', 'f', 'f', 'f', 'f', 'f', 'f', 'f', 'f', 'f', 'f', 'f', 'f', 'f', 'f', 'f', 'f', 'f', 'f', 'f', 'f', 'f', 'f', 'f', 'f', 'f', 'f', 'f', 'f', 'f', 'f', 'f', 'f', 'f', 'f', 'f', 'f', 'f', 'f', 'f', 'f', 'f', 'f', 'f', 'f', 'f', 'f', 'f', 'f', 'f', 'f', 'f', 'f', 'f', 'f', 'f', 'f', 'f', 'f', 'f', 'f', 'f', 'f', 'f', 'f', 'f', 'f', 'f', 'f', 'f', 'f', 'f', 'f', 'f', 'f', 'f', 'f', 'f', 'f', 'f', 'f', 'f', 'f', 'f', 'f', 'f', 'f', 'f', 'f', 'f', 'f', 'f', 'f', 'f', 'f', 'f', 'f', 'f', 'f', 'f', 'f', 'f', 'f', 'f', 'f', 'f', 'f', 'f', 'f', 'f', 'f', 'f', 'f', 'f', 'f', 'f', 'f', 'f', 'f', 'f', 'f', 'f', 'f', 'f', 'f', 'f', 'f', 'f', 'f', 'f', 'f', 'f', 'f', 'f', 'f', 'f', 'f', 'f', 'f', 'f', 'f', 'f', 'f', 'f', 'f', 'f', 'f', 'f', 'f', 'f', 'f', 'f', 'f', 'f', 'f', 'f', 'f', 'f', 'f', 'f', 'f', 'f', 'f', 'f', 'f', 'f', 'f', 'f', 'f', 'f', 'f', 'f', 'f', 'f', 'f', 'f', 'f', 'f', 'f', 'f', 'f', 'f', 'f', 'f', 'f', 'f', 'f', 'f', 'f', 'f', 'f', 'f', 'f', 'f', 'f', 'f', 'f', 'f', 'f', 'f', 'f', 'f', 'f', 'f', 'f', 'f', 'f', 'f', 'f', 'f', 'f', 'f', 'f', 'f', 'f', 'f', 'f', 'f', 'f', 'f', 'f', 'f', 'f', 'f', 'f', 'f', 'f', 'f', 'f', 'f', 'f', 'f', 'f', 'f', 'f', 'f', 'f', 'f', 'f', 'f', 'f', 'f', 'f', 'f', 'f', 'f', 'f', 'f', 'f', 'f', 'f', 'f', 'f', 'f', 'f', 'f', 'f', 'f', 'f', 'f', 'f', 'f', 'f', 'f', 'f', 'f', 'f', 'f', 'f', 'f', 'f', 'f', 'f', 'f', 'f', 'f', 'f', 'f', 'f', 'f', 'f', 'f', 'f', 'f', 'f', 'f', 'f', 'f', 'f', 'f', 'f', 'f', 'f', 'f', 'f', 'f', 'f', 'f', 'f', 'f', 'f', 'f', 'f', 'f', 'f', 'f', 'f', 'f', 'f', 'f', 'f', 'f', 'f', 'f', 'f', 'f', 'f', 'f', 'f', 'f', 'f', 'f', 'f', 'f', 'f', 'f', 'f', 'f', 'f', 'f', 'f', 'f', 'f', 'f', 'f', 'f', 'f', 'f', 'f', 'f', 'f', 'f', 'f', 'f', 'f', 'f', 'f', 'f', 'f', 'f', 'f', 'f', 'f', 'f', 'f', 'f', 'f', 'f', 'f', 'f', 'f', 'f', 'f', 'f', 'f', 'f', 'f', 'f', 'f', 'f', 'f', 'f', 'f', 'f', 'f', 'f', 'f', 'f', 'f', 'f', 'f', 'f', 'f', 'f', 'f', 'f', 'f', 'f', 'f', 'f', 'f', 'f', 'f', 'f', 'f', 'f', 'f', 'f', 'f', 'f', 'f', 'f', 'f', 'f', 'f', 'f', 'f', 'f', 'f', 'f', 'f', 'f', 'f', 'f', 'f', 'f', 'f', 'f', 'f', 'f', 'f', 'f', 'f', 'f', 'f', 'f', 'f', 'f', 'f', 'f', 'f', 'f', 'f', 'f', 'f', 'f', 'f', 'f', 'f', 'f', 'f', 'f', 'f', 'f', 'f', 'f', 'f', 'f', 'f', 'f', 'f', 'f', 'f', 'f', 'f', 'f', 'f', 'f', 'f', 'f', 'f', 'f', 'f', 'f', 'f', 'f', 'f', 'f', 'f', 'f', 'f', 'f', 'f', 'f', 'f', 'f', 'f', 'f', 'f', 'f', 'f', 'f', 'f', 'f', 'f', 'f', 'f', 'f', 'f', 'f', 'f', 'f', 'f', 'f', 'f', 'f', 'f', 'f', 'f', 'f', 'f', 'f', 'f', 'f', 'f', 'f', 'f', 'f', 'f', 'f', 'f', 'f', 'f', 'f', 'f', 'f', 'f', 'f', 'f', 'f', 'f', 'f', 'f', 'f', 'f', 'f', 'f', 'f', 'f', 'f', 'f', 'f', 'f', 'f', 'f', 'f', 'f', 'f', 'f', 'f', 'f', 'f', 'f', 'f', 'f', 'f', 'f', 'f', 'f', 'f', 'f', 'f', 'f', 'f', 'f', 'f', 'f', 'f', 'f', 'f', 'f', 'f', 'f', 'f', 'f', 'f', 'f', 'f', 'f', 'f', 'f', 'f', 'f', 'f', 'f', 'f', 'f', 'f', 'f', 'f', 'f', 'f', 'f', 'f', 'f', 'f', 'f', 'f', 'f', 'f', 'f', 'f', 'f', 'f', 'f', 'f', 'f', 'f', 'f', 'f', 'f', 'f', 'f', 'f', 'f', 'f', 'f', 'f', 'f', 'f', 'f', 'f', 'f', 'f', 'f', 'f', 'f', 'f', 'f', 'f', 'f', 'f', 'f', 'f', 'f', 'f', 'f', 'f', 'f', 'f', 'f', 'f', 'f', 'f', 'f', 'f', 'f', 'f', 'f', 'f', 'f', 'f', 'f', 'f', 'f', 'f', 'f', 'f', 'f', 'f', 'f', 'f', 'f', 'f', 'f', 'f', 'f', 'f', 'f', 'f', 'f', 'f', 'f', 'f', 'f', 'f', 'f', 'f', 'f', 'f', 'f', 'f', 'f', 'f', 'f', 'f', 'f', 'f', 'f', 'f', 'f', 'f', 'f', 'f', 'f', 'f', 'f', 'f', 'f', 'f', 'f', 'f', 'f', 'f', 'f', 'f', 'f', 'f', 'f', 'f', 'f', 'f', 'f', 'f', 'f', 'f', 'f', 'f', 'f', 'f', 'f', 'f', 'f', 'f', 'f', 'f', 'f', 'f', 'f', 'f', 'f', 'f', 'f', 'f', 'f', 'f', 'f', 'f', 'f', 'f', 'f', 'f', 'f', 'f', 'f', 'f', 'f', 'f', 'f', 'f', 'f', 'f', 'f', 'f', 'f', 'f', 'f', 'f', 'f', 'f', 'f', 'f', 'f', 'f', 'f', 'f', 'f', 'f', 'f', 'f', 'f', 'f', 'f', 'f', 'f', 'f', 'f', 'f', 'f', 'f', 'f', 'f', 'f', 'f', 'f', 'f', 'f', 'f', 'f', 'f', 'f', 'f', 'f', 'f', 'f', 'f', 'f', 'f', 'f', 'f', 'f', 'f', 'f', 'f', 'f', 'f', 'f', 'f', 'f', 'f', 'f', 'f', 'f', 'f', 'f', 'f', 'f', 'f', 'f', 'f', 'f', 'f', 'f', 'f', 'f', 'f', 'f', 'f', 'f', 'f', 'f', 'f', 'f', 'f', 'f', 'f', 'f', 'f', 'f', 'f', 'f', 'f', 'f', 'f', 'f', 'f', 'f', 'f', 'f', 'f', 'f', 'f', 'f', 'f', 'f', 'f', 'f', 'f', 'f', 'f', 'f', 'f', 'f', 'f', 'f', 'f', 'f', 'f', 'f', 'f', 'f', 'f', 'f', 'f', 'f', 'f', 'f', 'f', 'f', 'f', 'f', 'f', 'f', 'f', 'f', 'f', 'f', 'f', 'f', 'f', 'f', 'f', 'f', 'f', 'f', 'f', 'f', 'f', 'f', 'f', 'f', 'f', 'f', 'f', 'f', 'f', 'f', 'f');" ("object 3")
  n1 = String Subset(string=w10, offset (0)=64, length (rest)=49498 ("length (rest)")) -> (substring=w16:string)
  n2 = String Subset(string=w10, offset (0)=49574, length (rest)=7525 ("length (rest)")) -> (substring=w5:string)
  n3 = String Length(string="date/time string") -> (length=w4:i32)
  n4 = Add(x=w4, y=4) -> (x+y=w1:i32)
  n5 = Replace Substring(2:23 ("length (len. of substring)"), 3:1 ("offset (0)"), 4:"date/time string", 5:w5) -> (1:w37:string)  [unwired: 1 out]
  n6 = for {
    tunnel: "discret parameters" -> [w49] mode=indexing
    shift-right: [w51] -> w41
    shift-left: w37 -> [w53]
    shift-right: [w52] -> w9
    shift-left: w1 -> [w50]
    tunnel: "DI table" -> [w57] mode=indexing
    shift-right: [w56] -> w14
    shift-left: 1 -> [w54]
    shift-right: [w55] -> w20
    shift-left: w16 -> [w58]
    tunnel: "DI state table" -> [w48] mode=indexing
    shift-right: [w46] -> w6
    shift-left: FALSE -> [w45]
    n7 = Unbundle By Name(w48) -> ("code"=w47:i32)
    n8 = case shown="1, 9" w47 {
      tunnel: w58 -> [w63 w87]
      tunnel: w57 -> [_ w86]
      tunnel: [w61 w85] -> w56
      tunnel: [w63 w84] -> w55
      tunnel: w54 -> [w61 w83]
      tunnel: w53 -> [w62 w82]
      tunnel: [w60 w81] -> w52
      tunnel: [w62 w80] -> w51
      tunnel: w50 -> [w60 w79]
      tunnel: w49 -> [_ w78]
      tunnel: [w59 TRUE] -> w46
      tunnel: w45 -> [w59 _]
      frame 0, Default {
      }
      frame 1, 9 {
        w65 = 3 ("x+y")
        w72 = 2 ("x+y")
        w73 = 4 ("x+y")
        n9 = Select(t="'t'", s=w78, f="'f'") -> (s? t:f=w66:string)
        n10 = String Length(string=w86) -> (length=w77:i32)
        n11 = Add(x=w65, y=w79) -> (x+y=w69:i32)
        n12 = Replace Substring(2:w77, 3:w83, 4:w86, 5:w87) -> (1:w76:string)  [unwired: 1 out]
        n13 = Replace Substring(2:w65, 3:w79, 4:w66, 5:w82) -> (1:w70:string)  [unwired: 1 out]
        n14 = Add(x=w77, y=w83) -> (x+y=w74:i32)
        n15 = Add(x=w73, y=w74) -> (x+y=w85:i32)
        n16 = Add(x=w72, y=w69) -> (x+y=w81:i32)
        n17 = Replace Substring(2:w73, 3:w74, 4:"\", \" ", 5:w76) -> (1:w84:string)  [unwired: 1 out]
        n18 = Replace Substring(2:w72, 3:w69, 4:", ", 5:w70) -> (1:w80:string)  [unwired: 1 out]
      }
    }
  }
  "Data to write" <- w6
  n19 = Subtract(x=w14, y=3) -> (x-y=w13:i32)
  n20 = Subtract(x=w9, y=2) -> (x-y=w43:i32)
  n21 = Replace Substring(2:32 ("length (len. of substring)"), 3:w32, 4:"table", 5:w10) -> (1:w34:string)  [unwired: 1 out]
  n22 = String Subset(string=w20, length (rest)=w13) -> (substring=w24:string)  [unwired: 1 in]
  n23 = String Subset(string=w41, length (rest)=w43) -> (substring=w29:string)  [unwired: 1 in]
  n24 = String Length(string="table") -> (length=w31:i32)
  n25 = Compound Arithmetic op=ADD(w32, w31, 12 ("value")) -> (w28:i32)
  n26 = Replace Substring(2:49498 ("length (len. of substring)"), 3:w28, 4:w24, 5:w34) -> (1:w30:string)  [unwired: 1 out]
  n27 = String Length(string=w24) -> (length=w27:i32)
  n28 = Compound Arithmetic op=ADD(w28, w27, 11 ("value")) -> (w25:i32)
  n29 = Replace Substring(2:7526 ("length (len. of substring)"), 3:w25, 4:w29, 5:w30) -> (1:→"parameters":string)  [unwired: 1 out]
